vi "SpectrometerSpinCoater_v04_BetterStreaming.vi"() -> ()   [LabVIEW 2018]
uses:
  <instrlib>/Classes/CCD/Abstract_CCD/Abstract_CCD.lvclass
  TypDef/DeviceQueue_TypeDef.ctl
  TypDef/DeviceQueue_Action.ctl
  TypDef/DataQueue_TypeDef.ctl
  TypDef/DataQueue_Action.ctl
  <vilib>/Utility/error.llb/DialogType.ctl
  <instrlib>/Classes/CCD/Avantes/Avantes.lvclass
  C:/Program Files/National Instruments/LabVIEW 2018/instr.lib/Classes/CCD/Abstract_CCD/Abstract_CCD.lvclass
  <vilib>/Instr/_visa.llb/VISA Configure Serial Port (Instr).vi
panel:
  out "Time.spin":refnum<file>
  out "Meas.spin":refnum<file>
  out "Arduino":bool
  out "NKT":bool
  out "Spectromter":bool
  in  "Abort Button":bool
  in  "Stop Button":bool
  in  "Tab Control":enum32{"Measure", "Settings"}(tab)=enum."Settings"
  out "Action":string
  in  "Preview":bool
  out "XY Graph":T1(graph)
  in  "Frames for Dark/Ref":dbl=1.0
  in  "StartSpin_Button":bool
  out "Overall Time":dbl
  in  "Seconds after Spin Stop":dbl[unit]=0.5
  in  "Program Spin Coater\nSpeed (rpm)          Time (s)":dbl[][](array[numeric])
  in  "Record RefSpec":bool
  in  "Record_Darkspec":bool
  in  "Comments":string="Just for testing"
  in  "File Name":string="Temp"
  in  "Save Path":path=path "C:/Users/Timo/Desktop/SpinCoater/Measurement"
  in  "Seconds to Spin Start":dbl[unit]=1.0
  in  "Calculate Frames":bool=TRUE
  in  "Frames":i32
  out "Frame Rate":dbl[unit]
  in  "Integration Time":dbl[unit]=3e-05
  in  "StartMeasurement_Button":bool
  in  "Speed":dbl
  in  "Milliseconds":dbl
  in  "Debug":bool
  in  "Port Arduino":refnum<visa-resource-name>="COM6"
  out "Error Arduino":bool caption="Error"
  in  "Init_Arduino":bool=TRUE caption="Init"
  out "Caption_Settings_Arduino":string="Arduino"
  out "Caption_Settings_NKT":string="NKT Laser"
  out "Error_Spectromter":bool caption="Error"
  in  "Init_Spectrometer":bool=TRUE caption="Init"
  out "Caption_Settings_Spectrometer":string="Spectromter"
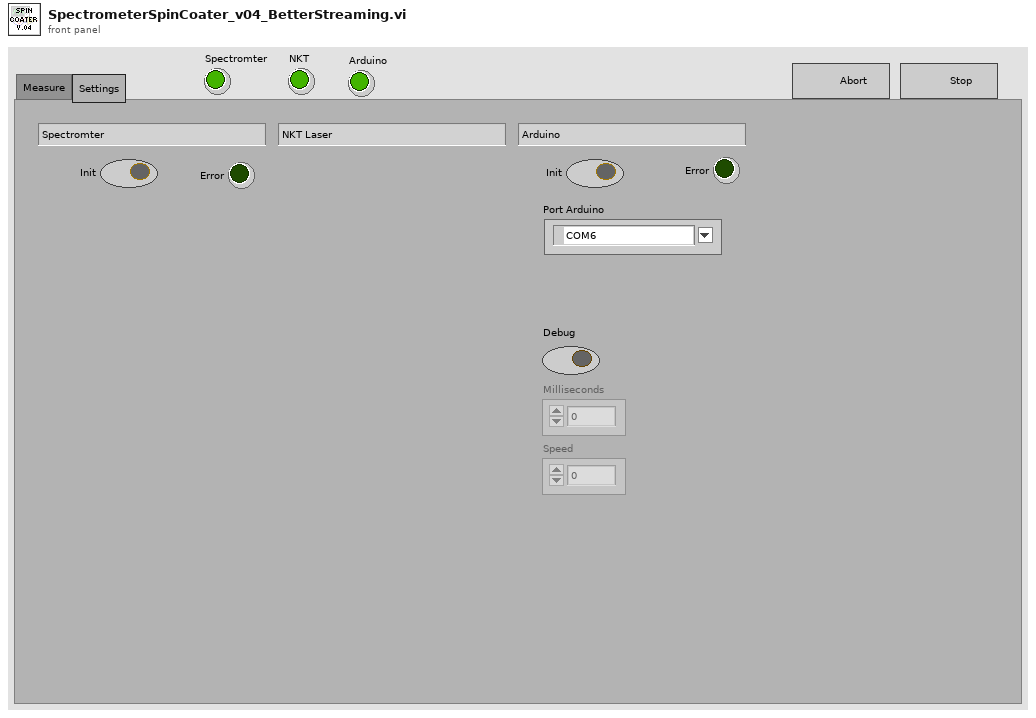
[diagram p1: front panel]
types:
  T1 = cluster{"Wavlength":dbl[unit][], "Image":dbl[]}[]
  T2 = cluster{"Dark":cluster{"Image":dbl[][][], "Frame Size":cluster{"F":i32, "Y":i32, "X":i32}}[], "Ref":cluster{"Image":dbl[][][], "Frame Size":cluster{"F":i32, "Y":i32, "X":i32}}[], "Wavlength":dbl[unit][], "spec":dbl[][]}
  T3 = cluster{"Port Arduino":refnum<visa-resource-name>, "Abstract_CCD.lvclass":refnum<class "Abstract_CCD.lvclass">}
  T4 = typedef "DataQueue_TypeDef.ctl" = cluster{"QueueAction":T5, "Data":cluster{"Image":dbl[][][], "Frame Size":cluster{"F":i32, "Y":i32, "X":i32}}[], "Data_Raw":cluster{"Image":dbl[][][], "Frame Size":cluster{"F":i32, "Y":i32, "X":i32}}[], "Data_Dark":cluster{"Image":dbl[][][], "Frame Size":cluster{"F":i32, "Y":i32, "X":i32}}[], "Data_Ref":cluster{"Image":dbl[][][], "Frame Size":cluster{"F":i32, "Y":i32, "X":i32}}[], "Device Information":string[], "Numeric Control":dbl, "Boolean":bool, "Wavelength":dbl[unit][], "Time":dbl[], "Time Stamp":timestamp, "Numeric Control 2":dbl}
  T5 = typedef "DataQueue_Action.ctl" = enum16{"TimeOut", "Close_Program", "Stop_Measurement", "Measure_InSituSpinCoating", "Save_Data", "Set_Ref", "Set_Dark", "Set_Wavelength", "Spectrometer_Measure", "Transfer_Settings"}
  T6 = typedef "DeviceQueue_TypeDef.ctl" = cluster{"QueueAction":T7, "Numeric 1":dbl, "Numeric 2":dbl, "Boolean 1":bool, "Boolean 2":bool, "Spin Program":dbl[][]}
  T7 = typedef "DeviceQueue_Action.ctl" = enum16{"TimeOut", "Close_Program", "Abort", "Spectrometer_Init", "Spectrometer_Close", "Spectrometer_DeviceInformation", "Spectrometer_Measure", "Spectrometer_Preview", "Spectrometer_Abort", "Spectrometer_StartMeasurement", "Spectrometer_GetData", "Spectrometer_StopMeasurement", "Spectrometer_SetIntegrationTime", "Spectrometer_SetFrames", "Spectrometer_SetDarkspec", "Spectrometer_SetReference", "Spectrometer_SetTriggerMode", "Laser_Init", "Laser_Close", "Arduino_Init", "Arduino_Close", "Arduino_LoadProgram", "Arduino_StartProgram", "Arduino_SetSpeed", "Arduino_SetMillis", "Arduino_StopSpin", "Measure_InSitu", "Measure_Stop"}
  T8 = enum16{"open", "replace", "create", "open or create", "replace or create", "replace or create with confirmation"}
  T9 = cluster{"Image":dbl[][][], "Frame Size":cluster{"F":i32, "Y":i32, "X":i32}}[]
  T10 = cluster{"Image":dbl[][][], "Frame Size":cluster{"F":i32, "Y":i32, "X":i32}}
  T11 = cluster{"Image":dbl[], "Image":dbl[], dbl[], "Numeric Control":dbl, "Numeric Control 2":dbl}
  T12 = typedef "DialogType.ctl" = u16
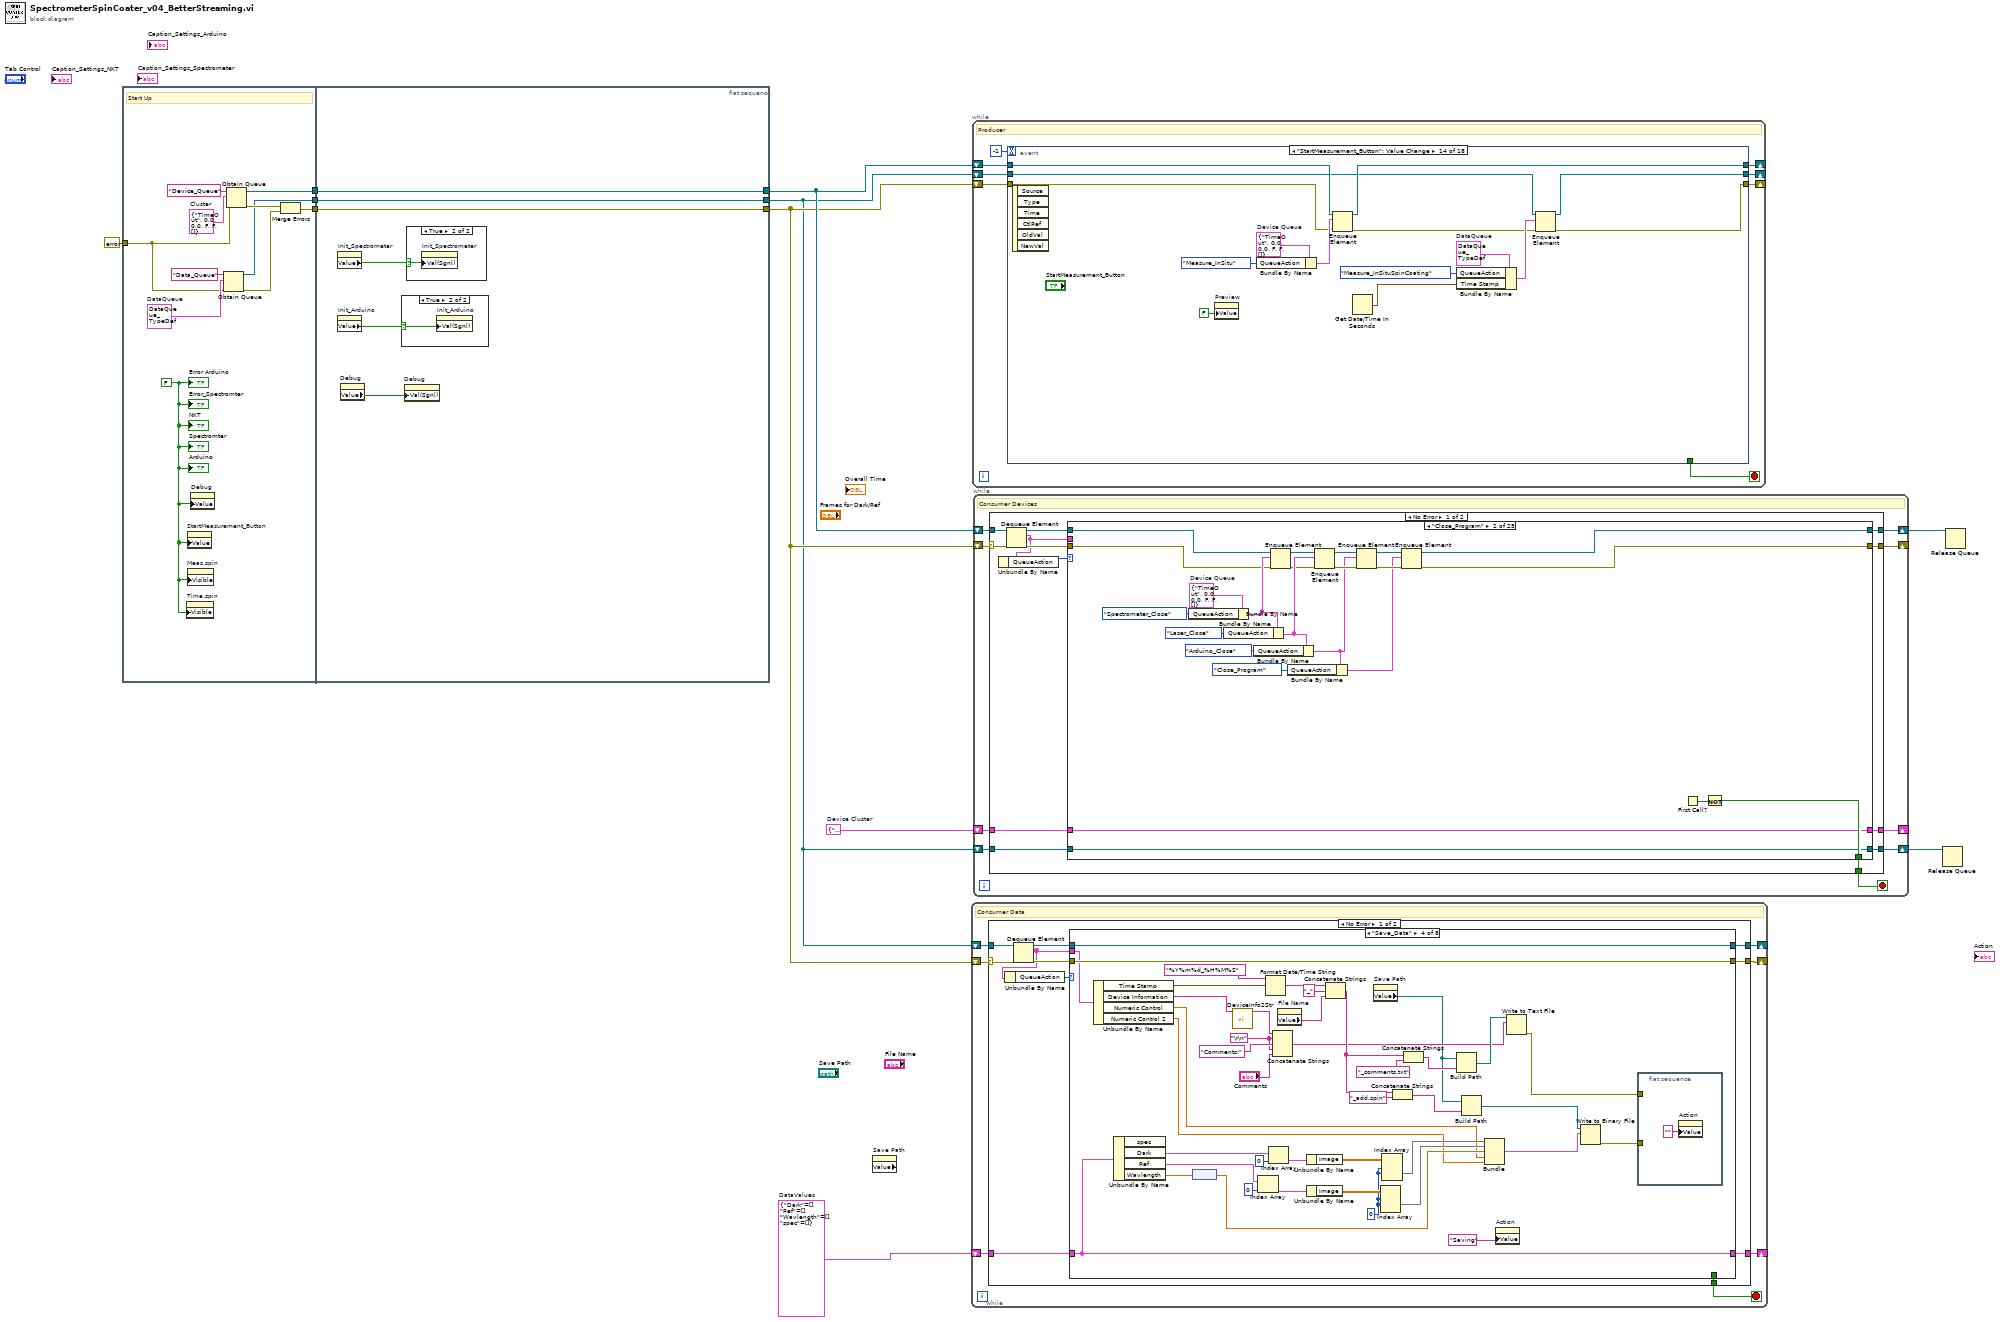
[diagram p0: block diagram]
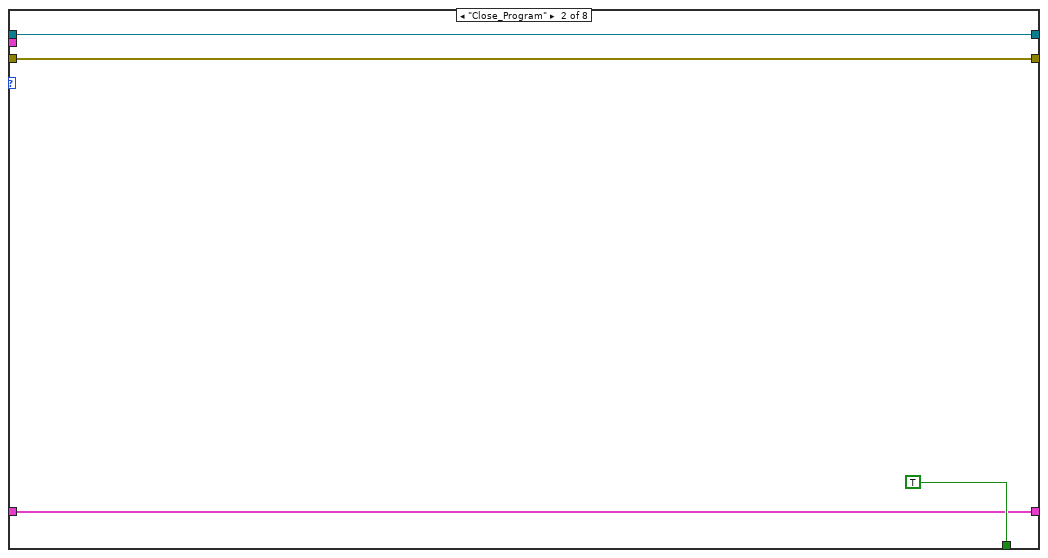
[diagram p5: hidden frame]
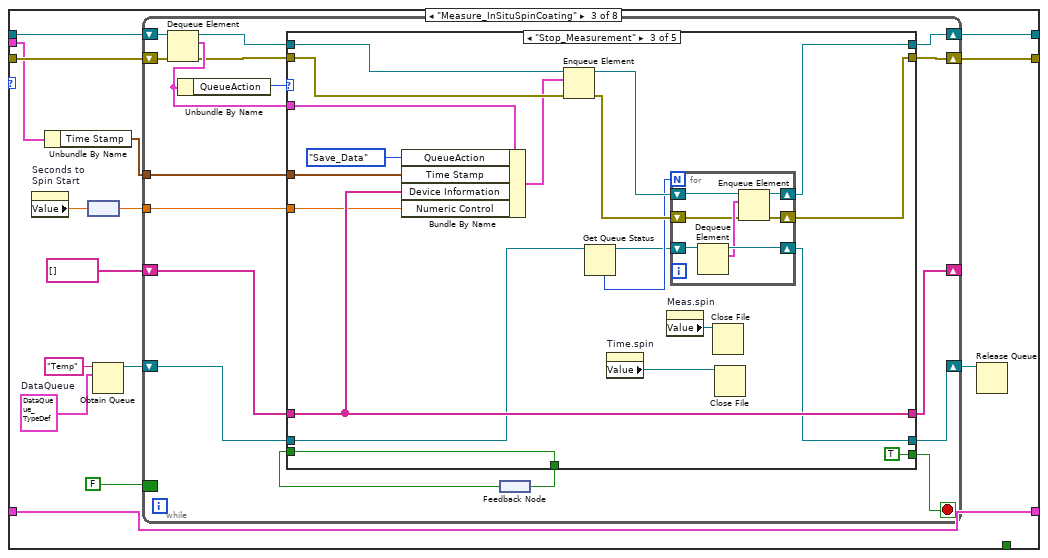
[diagram p6: hidden frame]
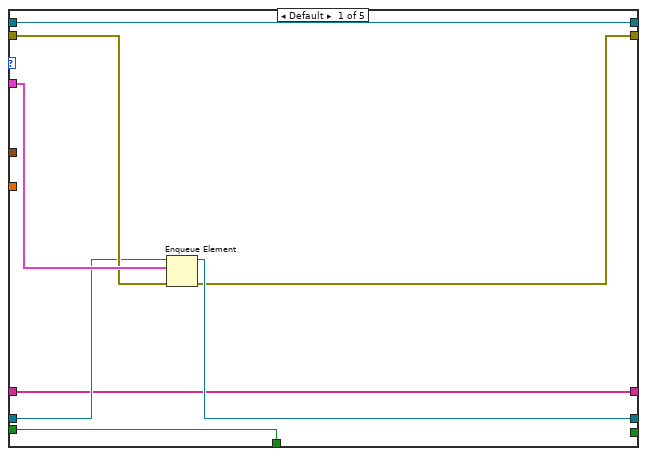
[diagram p7: hidden frame]
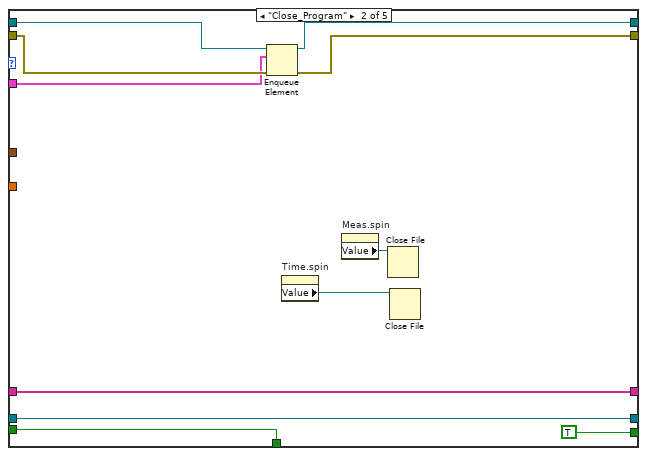
[diagram p8: hidden frame]
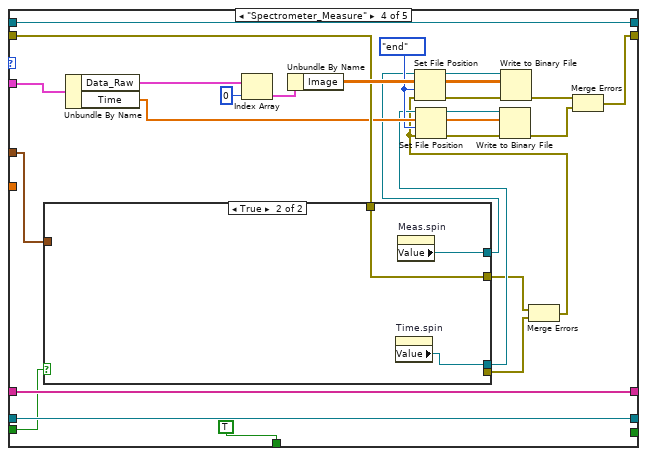
[diagram p9: hidden frame]
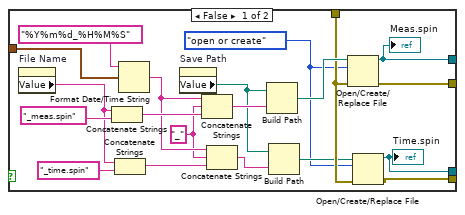
[diagram p10: hidden frame]
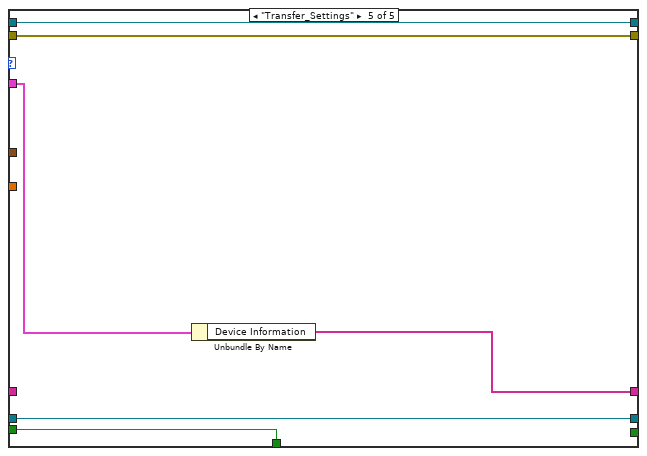
[diagram p11: hidden frame]
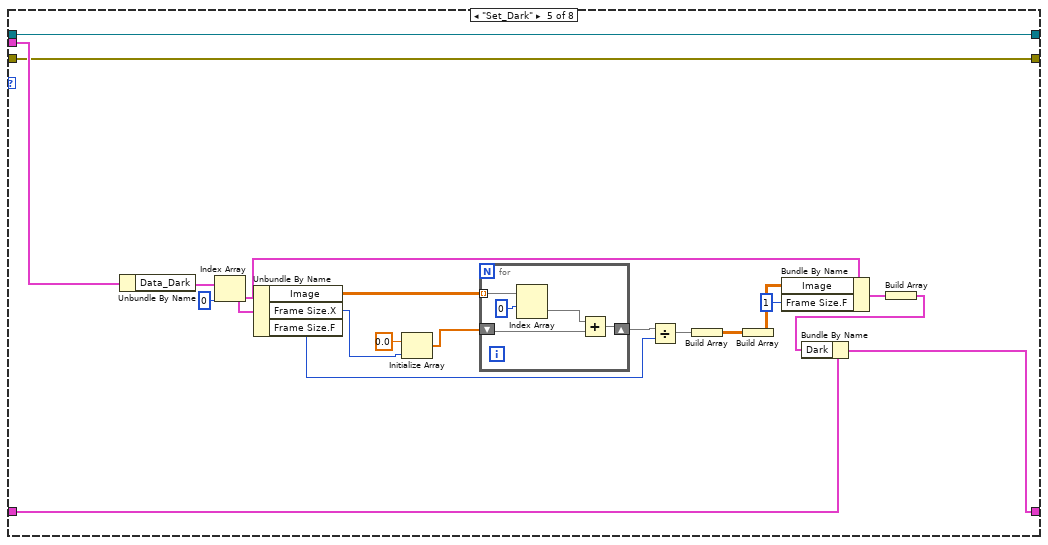
[diagram p12: hidden frame]
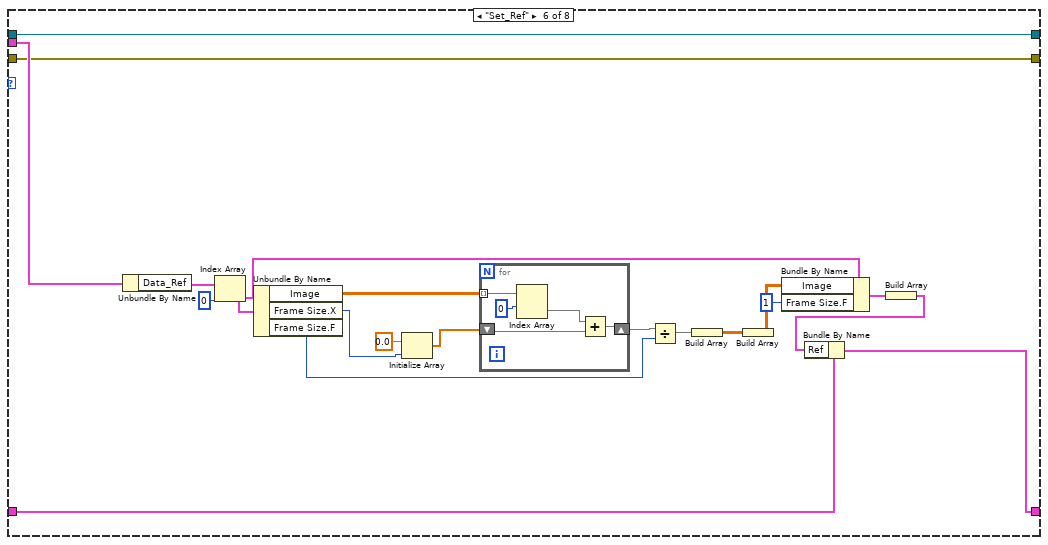
[diagram p13: hidden frame]
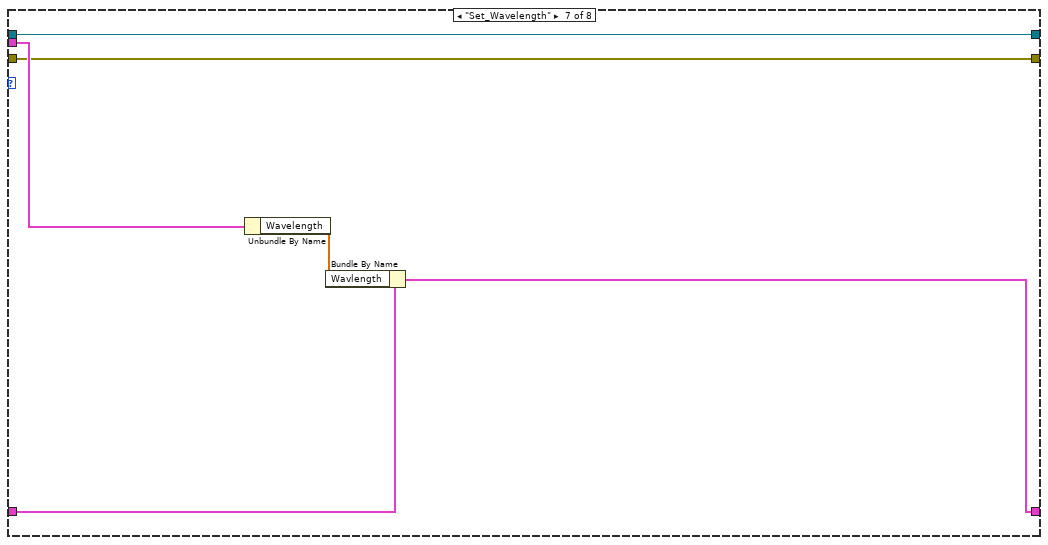
[diagram p14: hidden frame]
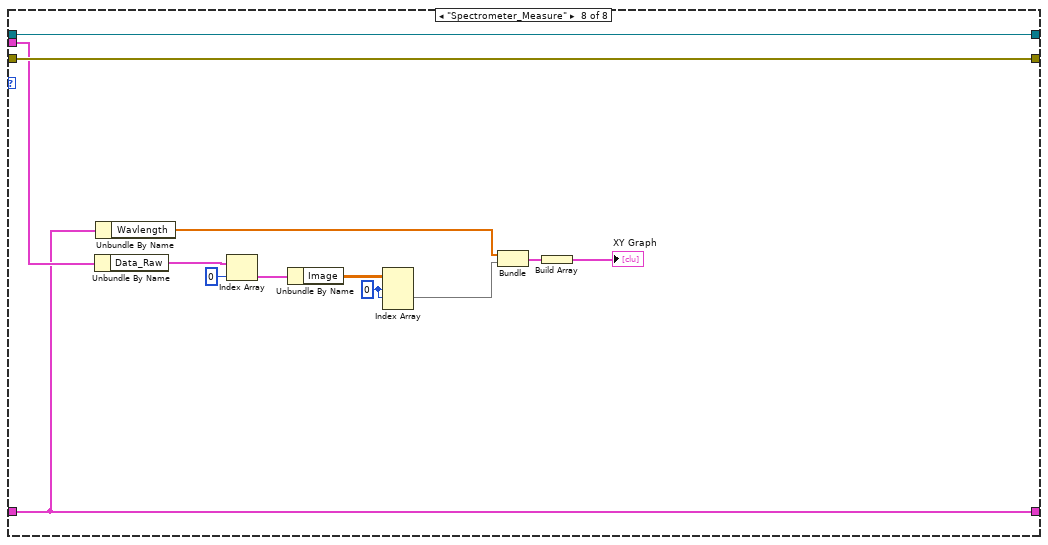
[diagram p15: hidden frame]
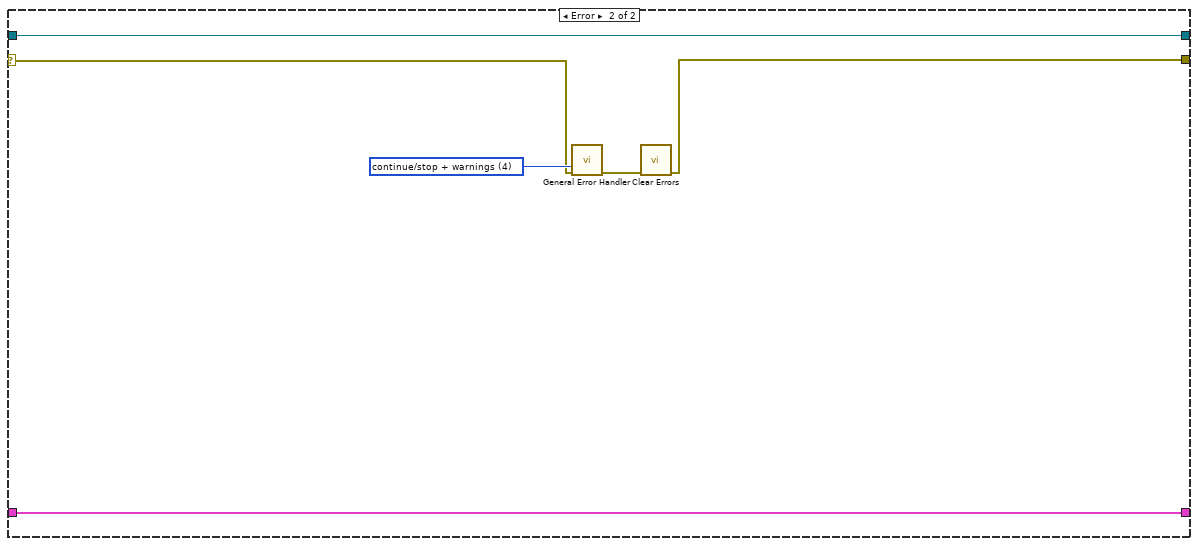
[diagram p16: hidden frame]
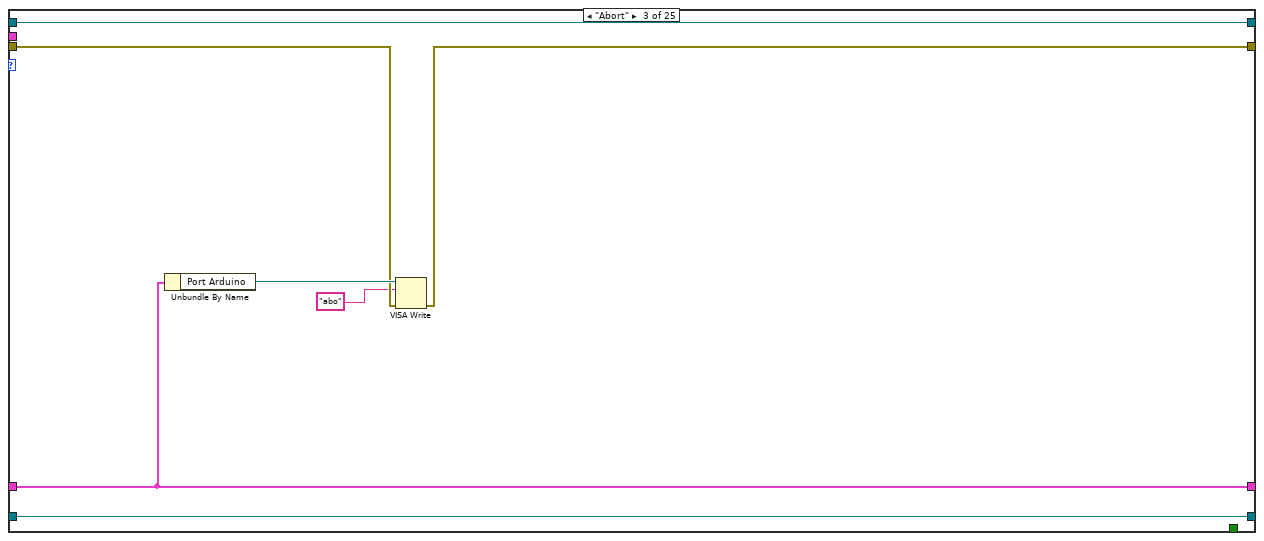
[diagram p18: hidden frame]
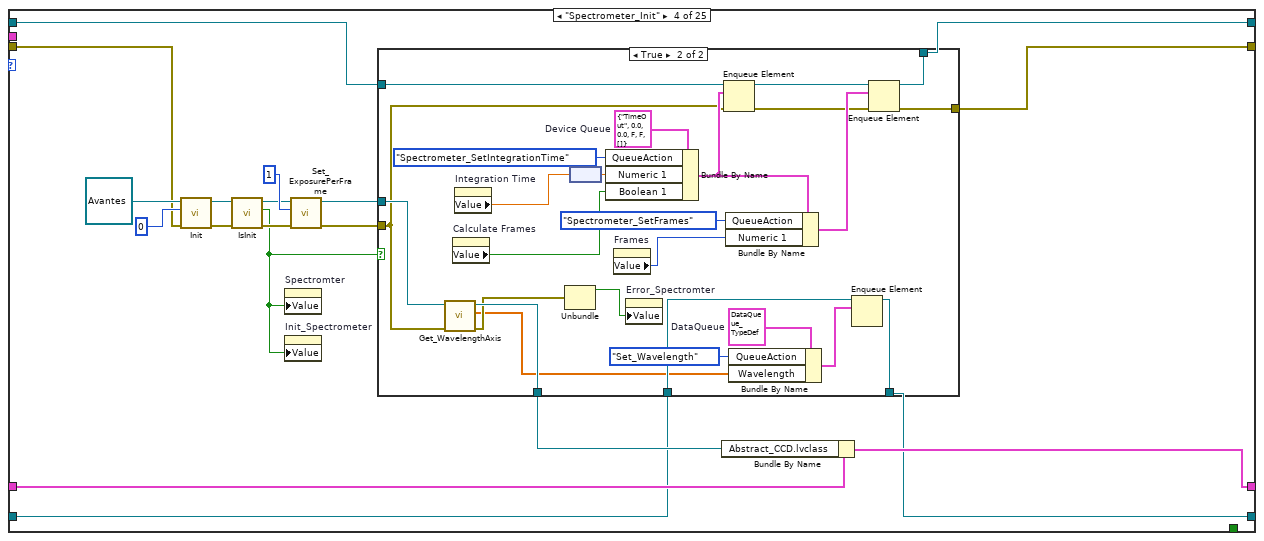
[diagram p19: hidden frame]
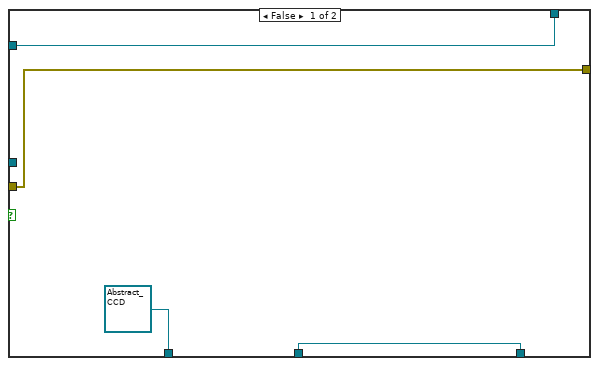
[diagram p20: hidden frame]
diagram:
  w1 = T2 {"Dark"=[], "Ref"=[], "Wavlength"=[], "spec"=[]}  # DataValues
  w6 = T3 {"Port Arduino"="", "Abstract_CCD.lvclass"=refnum}  # Device Cluster
  n1 = flat-sequence {
    tunnel: errorcluster {"status"=FALSE, "code"=0, "source"=""} ("error constant") -> [w17]
    tunnel: [w20] -> w10
    tunnel: [w14] -> w9
    tunnel: [w13] -> w8
    tunnel: w10 -> [w26]
    tunnel: w9 -> [w25]
    tunnel: w8 -> [w24]
    tunnel: [w26] -> w7
    tunnel: [w25] -> w2
    tunnel: [w24] -> w3
    frame #0 {
      w18 = T4 {"QueueAction"=enum."TimeOut", "Data"=[], "Data_Raw"=[], "Data_Dark"=[], "Data_Ref"=[], "Device Information"=[], "Numeric Control"=0.0, "Boolean"=FALSE, "Wavelength"=[], "Time"=[], "Time Stamp"=timestamp(0 s since 1904-01-01), "Numeric Control 2"=0.0}  # DataQueue
      w21 = T6 {"QueueAction"=enum."TimeOut", "Numeric 1"=0.0, "Numeric 2"=0.0, "Boolean 1"=FALSE, "Boolean 2"=FALSE, "Spin Program"=[]}  # Cluster
      w12 = FALSE ("Error Arduino")
      # "Start Up"
      n2 = property on="Time.spin" class="Ref (strict)"("Visible"=w12) -> ()  [unwired: 2 in, 2 out]
      n3 = property on="StartMeasurement_Button" class="Bool (strict)"("Value"=w12) -> ()  [unwired: 2 in, 2 out]
      n4 = property on="Meas.spin" class="Ref (strict)"("Visible"=w12) -> ()  [unwired: 2 in, 2 out]
      n5 = property on="Debug" class="Bool (strict)"("Value"=w12) -> ()  [unwired: 2 in, 2 out]
      n6 = Obtain Queue(name (unnamed)="Data_Queue", element data type=w18, error in (no error)=w17) -> (queue out=w14:refnum<queue>, error out=w15:errorcluster)  [unwired: 2 in, 1 out]
      n7 = Obtain Queue(name (unnamed)="Device_Queue", element data type=w21, error in (no error)=w17) -> (queue out=w20:refnum<queue>, error out=w16:errorcluster)  [unwired: 2 in, 1 out]
      n8 = Merge Errors(w16, w15) -> (w13:errorcluster)
      "Error_Spectromter" <- w12
      "Error Arduino" <- w12
      "Spectromter" <- w12
      "NKT" <- w12
      "Arduino" <- w12
    }
    frame #1 {
      n9 = property on="Init_Spectrometer" class="Bool (strict)"() -> ("Value"=w28:bool)  [unwired: 2 in, 2 out]
      n10 = property on="Init_Arduino" class="Bool (strict)"() -> ("Value"=w27:bool)  [unwired: 2 in, 2 out]
      n11 = property on="Debug" class="Bool (strict)"() -> ("Value"=w23:bool)  [unwired: 2 in, 2 out]
      n12 = case shown="True" w27 {
        selector: w27 -> [_ w29]
        frame False {
        }
        frame True {
          n13 = property on="Init_Arduino" class="Bool (strict)"("Val(Sgnl)"=w29) -> ()  [unwired: 2 in, 2 out]
        }
      }
      n14 = property on="Debug" class="Bool (strict)"("Val(Sgnl)"=w23) -> ()  [unwired: 2 in, 2 out]
      n15 = case shown="True" w28 {
        selector: w28 -> [_ w30]
        frame False {
        }
        frame True {
          n16 = property on="Init_Spectrometer" class="Bool (strict)"("Val(Sgnl)"=w30) -> ()  [unwired: 2 in, 2 out]
        }
      }
    }
  }
  n17 = property on="Save Path" class="Path" props=["Value"]() -> ()  [unwired: 2 in, 3 out]
  n18 = while {
    shift-right: [w31] -> _
    shift-left: w3 -> [w37]
    shift-right: [w32] -> _
    shift-left: w2 -> [w36]
    shift-right: [w33] -> _
    shift-left: w1 -> [w35]
    stop <- w34 stop-if-true
    # "Consumer Data"
    n19 = case shown="No Error" w37 {
      selector: w37 -> [w48 w303]
      tunnel: w36 -> [w47 w304]
      tunnel: w35 -> [w45 w301]
      tunnel: [w44 _] -> w34
      tunnel: [w43 w301] -> w33
      tunnel: [w42 w304] -> w32
      tunnel: [w40 w302] -> w31
      frame No Error {
        n20 = Dequeue Element(queue=w47, error in (no error)=w48) -> (queue out=w41:refnum<queue>, element=w38:T4, error out=w39:errorcluster)  [unwired: 1 in, 1 out]
        n21 = Unbundle By Name(w38) -> ("QueueAction"=w46:T5)
        n22 = case shown="\"Save_Data\"" w46 {
          tunnel: w45 -> [w49 w54 w60 w199 w251 w276 w286 w297]
          tunnel: [_ TRUE _ _ _ _ _ _] -> w44
          tunnel: [w49 w54 w60 w199 w247 w272 w285 w297] -> w43
          tunnel: [w51 w53 w70 w230 w248 w273 w282 w300] -> w42
          tunnel: w41 -> [w51 w53 w68 w230 w248 w273 w282 w300]
          tunnel: [w50 w52 w69 w229 w249 w274 w283 w299] -> w40
          tunnel: w39 -> [w50 w52 w67 w229 w249 w274 w283 w299]
          tunnel: w38 -> [_ _ w62 w215 w250 w275 w284 w298]
          frame "TimeOut", Default {
          }
          frame "Close_Program" {
          }
          frame "Measure_InSituSpinCoating" {
            w65 = T4 {"QueueAction"=enum."TimeOut", "Data"=[], "Data_Raw"=[], "Data_Dark"=[], "Data_Ref"=[], "Device Information"=[], "Numeric Control"=0.0, "Boolean"=FALSE, "Wavelength"=[], "Time"=[], "Time Stamp"=timestamp(0 s since 1904-01-01), "Numeric Control 2"=0.0}  # DataQueue
            n23 = property on="Seconds to\nSpin Start" class="DigNum (strict)"() -> ("Value"=w57:dbl[unit])  [unwired: 2 in, 2 out]
            n24 = Unbundle By Name(w62) -> ("Time Stamp"=w61:timestamp)
            n25 = node(w57) -> (w56:dbl)
            n26 = Obtain Queue(name (unnamed)="Temp", element data type=w65) -> (queue out=w64:refnum<queue>)  [unwired: 3 in, 2 out]
            n27 = while {
              shift-right: [w78] -> w70
              shift-left: w68 -> [w87]
              shift-right: [w79] -> w69
              shift-left: w67 -> [w86]
              shift-right: [w80] -> w63
              shift-left: w64 -> [w81]
              tunnel: w61 -> [w74]
              shift-right: [w75] -> _
              shift-left: string[] [] ("Device Information") -> [w76]
              border: FALSE -> [_]
              tunnel: w56 -> [w71]
              stop <- w77 stop-if-true
              n28 = Dequeue Element(queue=w87, error in (no error)=w86) -> (queue out=w82:refnum<queue>, element=w84:T4, error out=w83:errorcluster)  [unwired: 1 in, 1 out]
              n29 = Unbundle By Name(w84) -> ("QueueAction"=w85:T5)
              n30 = feedback #1() -> (w73:bool)
              n31 = case shown="\"Stop_Measurement\"" w85 {
                tunnel: w84 -> [w95 w104 w125 w158 w187]
                tunnel: w83 -> [w94 w105 w122 w148 w184]
                tunnel: w82 -> [w90 w106 w121 w157 w185]
                tunnel: w81 -> [w93 w101 w116 w145 w188]
                tunnel: [w92 w101 w113 w145 w188] -> w80
                tunnel: [w91 w102 w112 w146 w184] -> w79
                tunnel: [w90 w103 w111 w157 w185] -> w78
                tunnel: [_ TRUE TRUE _ _] -> w77
                tunnel: w76 -> [w89 w99 w123 w143 _]
                tunnel: [w89 w99 w123 w143 w186] -> w75
                tunnel: w74 -> [_ _ w124 w159 _]
                tunnel: w73 -> [w88 w98 w110 w141 w183]
                tunnel: [w88 w98 w110 TRUE w183] -> w72
                tunnel: w71 -> [_ _ w107 _ _]
                frame Default {
                  n32 = Enqueue Element(queue=w93, element=w95, error in (no error)=w94) -> (queue out=w92:refnum<queue>, error out=w91:errorcluster)  [unwired: 1 in, 1 out]
                }
                frame "Close_Program" {
                  n33 = Enqueue Element(queue=w106, element=w104, error in (no error)=w105) -> (queue out=w103:refnum<queue>, error out=w102:errorcluster)  [unwired: 1 in, 1 out]
                  n34 = property on="Time.spin" class="Ref (strict)"() -> ("Value"=w96:refnum<file>)  [unwired: 2 in, 2 out]
                  n35 = property on="Meas.spin" class="Ref (strict)"() -> ("Value"=w97:refnum<file>)  [unwired: 2 in, 2 out]
                  n36 = Close File(refnum=w97) -> ()  [unwired: 1 in, 2 out]
                  n37 = Close File(refnum=w96) -> ()  [unwired: 1 in, 2 out]
                }
                frame "Stop_Measurement" {
                  n38 = Bundle By Name(cluster=w125, "QueueAction"=DataQueue_Action."Save_Data", "Time Stamp"=w124, "Device Information"=w123, "Numeric Control"=w107) -> (w120:T4)
                  n39 = Enqueue Element(queue=w121, element=w120, error in (no error)=w122) -> (queue out=w118:refnum<queue>, error out=w117:errorcluster)  [unwired: 1 in, 1 out]
                  n40 = Get Queue Status(queue=w116) -> (queue out=w114:refnum<queue>, # elements in queue=w115:i32)  [unwired: 2 in, 6 out]
                  n41 = property on="Time.spin" class="Ref (strict)"() -> ("Value"=w108:refnum<file>)  [unwired: 2 in, 2 out]
                  n42 = property on="Meas.spin" class="Ref (strict)"() -> ("Value"=w109:refnum<file>)  [unwired: 2 in, 2 out]
                  n43 = for {
                    N: w115 -> [_]
                    shift-right: [w132] -> w113
                    shift-left: w114 -> [w133]
                    shift-right: [w129] -> w111
                    shift-left: w118 -> [w130]
                    shift-right: [w127] -> w112
                    shift-left: w117 -> [w128]
                    n44 = Dequeue Element(queue=w133) -> (queue out=w132:refnum<queue>, element=w131:T4)  [unwired: 2 in, 2 out]
                    n45 = Enqueue Element(queue=w130, element=w131, error in (no error)=w128) -> (queue out=w129:refnum<queue>, error out=w127:errorcluster)  [unwired: 1 in, 1 out]
                  }
                  n46 = Close File(refnum=w109) -> ()  [unwired: 1 in, 2 out]
                  n47 = Close File(refnum=w108) -> ()  [unwired: 1 in, 2 out]
                }
                frame "Spectrometer_Measure" {
                  w144 = enum16{"start", "end", "current"}."end" ("from (0:start)")
                  n48 = case shown="True" w141 {
                    tunnel: w159 -> [w176 _]
                    tunnel: w148 -> [w171 w182]
                    tunnel: [w164 w182] -> w135
                    tunnel: [w163 _] -> w136
                    tunnel: [w162 w181] -> w138
                    tunnel: [w161 w180] -> w137
                    frame False {
                      w165 = T8."open or create" ("operation (0:open)")
                      w160 = "_" ("string")
                      n49 = property on="File Name" class="Str"() -> ("Value"=w174:string)  [unwired: 2 in, 2 out]
                      n50 = Concatenate Strings(w174, "_meas.spin" ("string")) -> (w177:string)
                      n51 = Concatenate Strings(w174, "_time.spin" ("string")) -> (w169:string)
                      n52 = Format Date/Time String(time format string (%c)="%Y%m%d_%H%M%S", seconds (now)=w176) -> (date/time string=w170:string)  [unwired: 1 in]
                      n53 = property on="Save Path" class="Path"() -> ("Value"=w167:path)  [unwired: 2 in, 2 out]
                      n54 = Concatenate Strings(w170, w160, w177) -> (w175:string)
                      n55 = Concatenate Strings(w170, w160, w169) -> (w168:string)
                      n56 = Build Path(base path=w167, name or relative path=w175) -> (appended path=w172:path)
                      n57 = Build Path(base path=w167, name or relative path=w168) -> (appended path=w166:path)
                      n58 = Open/Create/Replace File(file path (use dialog)=w172, error in=w171, operation (0:open)=w165) -> (refnum out=w162:refnum<file>, error out=w164:errorcluster)  [unwired: 3 in, 1 out]
                      "Meas.spin" <- w162
                      n59 = Open/Create/Replace File(file path (use dialog)=w166, error in=w171, operation (0:open)=w165) -> (refnum out=w161:refnum<file>, error out=w163:errorcluster)  [unwired: 3 in, 1 out]
                      "Time.spin" <- w161
                    }
                    frame True {
                      n60 = property on="Time.spin" class="Ref (strict)"() -> ("Value"=w180:refnum<file>)  [unwired: 2 in, 2 out]
                      n61 = property on="Meas.spin" class="Ref (strict)"() -> ("Value"=w181:refnum<file>)  [unwired: 2 in, 2 out]
                    }
                  }
                  n62 = Unbundle By Name(w158) -> ("Data_Raw"=w154:T9, "Time"=w147:dbl[])
                  n63 = Index Array(array=w154, index=0) -> (element=w153:T10)
                  n64 = Unbundle By Name(w153) -> ("Image"=w151:dbl[][][])
                  n65 = Merge Errors(w135, w136) -> (w134:errorcluster)
                  n66 = Set File Position(refnum=w138, from (0:start)=w144, error in=w134) -> (refnum out=w150:refnum<file>, error out=w149:errorcluster)  [unwired: 1 in]
                  n67 = Set File Position(refnum=w137, from (0:start)=w144, error in=w134) -> (refnum out=w156:refnum<file>, error out=w155:errorcluster)  [unwired: 1 in]
                  n68 = Write to Binary File(file (use dialog)=w156, data=w147, error in=w155) -> (error out=w139:errorcluster)  [unwired: 3 in, 2 out]
                  n69 = Write to Binary File(file (use dialog)=w150, data=w151, error in=w149) -> (error out=w140:errorcluster)  [unwired: 3 in, 2 out]
                  n70 = Merge Errors(w140, w139) -> (w146:errorcluster)
                }
                frame "Transfer_Settings" {
                  n71 = Unbundle By Name(w187) -> ("Device Information"=w186:string[])
                }
              }
              n72 = feedback-in #1(w72) -> ()
            }
            n73 = Release Queue(queue=w63) -> ()  [unwired: 2 in, 3 out]
          }
          frame "Save_Data" {
            w201 = "\r\n"
            w219 = 0 ("index (page)")
            n74 = Unbundle By Name(w215) -> ("Time Stamp"=w213:timestamp, "Device Information"=w204:string[], "Numeric Control"=w198:dbl, "Numeric Control 2"=w197:dbl)
            n75 = Unbundle By Name(w199) -> ("Dark"=w226:T9, "Ref"=w224:T9, "Wavlength"=w228:dbl[unit][])  [unwired: 1 out]
            n76 = node(w228) -> (w216:dbl[])
            n77 = call "DeviceInfo2Str.vi"("Device Information"=w204) -> ("String"=w203:string)  [unwired: 10 in]
            n78 = Index Array(array=w224, index=0) -> (element=w222:T10)
            n79 = Format Date/Time String(time format string (%c)="%Y%m%d_%H%M%S", seconds (now)=w213) -> (date/time string=w212:string)  [unwired: 1 in]
            n80 = Index Array(array=w226, index=0) -> (element=w223:T10)
            n81 = Concatenate Strings(w203, w201, "Comments:" ("string"), w201, "Comments") -> (w196:string)
            n82 = property on="File Name" class="Str"() -> ("Value"=w194:string)  [unwired: 2 in, 2 out]
            n83 = Unbundle By Name(w223) -> ("Image"=w221:dbl[][][])
            n84 = Unbundle By Name(w222) -> ("Image"=w220:dbl[][][])
            n85 = Concatenate Strings(w212, "_" ("string"), w194) -> (w210:string)
            n86 = property on="Save Path" class="Path"() -> ("Value"=w193:path)  [unwired: 2 in, 2 out]
            n87 = Index Array(array=w220, index (dim 0)=w219, index (dim 1)=w219) -> (element=w217:dbl[])  [unwired: 1 in]
            n88 = Index Array(array=w221, index (dim 0)=w219, index (dim 1)=w219) -> (element=w218:dbl[])  [unwired: 1 in]
            n89 = Concatenate Strings(w210, "_add.spin" ("string")) -> (w208:string)
            n90 = Concatenate Strings(w210, "_comments.txt" ("string")) -> (w207:string)
            n91 = Build Path(base path=w193, name or relative path=w207) -> (appended path=w206:path)
            n92 = Build Path(base path=w193, name or relative path=w208) -> (appended path=w192:path)
            n93 = Bundle("Image"=w218, "Image"=w217, w216, "Numeric Control"=w198, "Numeric Control 2"=w197) -> (w191:T11)  [unwired: 1 in]
            n94 = property on="Action" class="Str"("Value"="Saving" ("Action")) -> ()  [unwired: 2 in, 2 out]
            n95 = Write to Text File(file (use dialog)=w206, text=w196) -> (error out=w190:errorcluster)  [unwired: 2 in, 2 out]
            n96 = Write to Binary File(file (use dialog)=w192, data=w191) -> (error out=w189:errorcluster)  [unwired: 4 in, 2 out]
            n97 = flat-sequence {
              tunnel: w190 -> [_]
              tunnel: w189 -> [_]
              frame #0 {
                n98 = property on="Action" class="Str"("Value"="" ("Action")) -> ()  [unwired: 2 in, 2 out]
              }
            }
          }
          frame "Set_Dark" {
            n99 = Unbundle By Name(w250) -> ("Data_Dark"=w237:T9)
            n100 = Index Array(array=w237, index=0) -> (element=w236:T10)
            n101 = Unbundle By Name(w236) -> ("Image"=w245:dbl[][][], "Frame Size.X"=w243:i32, "Frame Size.F"=w240:i32)
            n102 = Initialize Array(0.0 ("element"), w243) -> (w242:dbl[])
            n103 = for {
              tunnel: w245 -> [w256] mode=indexing
              shift-right: [w252] -> w241
              shift-left: w242 -> [w253]
              n104 = Index Array(array=w256, index (row)=0) -> (element=w254:dbl[])  [unwired: 1 in]
              n105 = Add(x=w254, y=w253) -> (x+y=w252:dbl[])
            }
            n106 = Divide(x=w241, y=w240) -> (x/y=w239:dbl[])
            n107 = Build Array(w239) -> (w238:dbl[][])
            n108 = Build Array(w238) -> (w235:dbl[][][])
            n109 = Bundle By Name(cluster=w236, "Image"=w235, "Frame Size.F"=1) -> (w233:T10)
            n110 = Build Array(w233) -> (w232:T9)
            n111 = Bundle By Name(cluster=w251, "Dark"=w232) -> (w247:T2)
          }
          frame "Set_Ref" {
            n112 = Unbundle By Name(w275) -> ("Data_Ref"=w262:T9)
            n113 = Index Array(array=w262, index=0) -> (element=w261:T10)
            n114 = Unbundle By Name(w261) -> ("Image"=w270:dbl[][][], "Frame Size.X"=w268:i32, "Frame Size.F"=w265:i32)
            n115 = Initialize Array(0.0 ("element"), w268) -> (w267:dbl[])
            n116 = for {
              tunnel: w270 -> [w281] mode=indexing
              shift-right: [w277] -> w266
              shift-left: w267 -> [w278]
              n117 = Index Array(array=w281, index (row)=0) -> (element=w279:dbl[])  [unwired: 1 in]
              n118 = Add(x=w279, y=w278) -> (x+y=w277:dbl[])
            }
            n119 = Divide(x=w266, y=w265) -> (x/y=w264:dbl[])
            n120 = Build Array(w264) -> (w263:dbl[][])
            n121 = Build Array(w263) -> (w260:dbl[][][])
            n122 = Bundle By Name(cluster=w261, "Image"=w260, "Frame Size.F"=1) -> (w258:T10)
            n123 = Build Array(w258) -> (w257:T9)
            n124 = Bundle By Name(cluster=w276, "Ref"=w257) -> (w272:T2)
          }
          frame "Set_Wavelength" {
            n125 = Unbundle By Name(w284) -> ("Wavelength"=w287:dbl[unit][])
            n126 = Bundle By Name(cluster=w286, "Wavlength"=w287) -> (w285:T2)
          }
          frame "Spectrometer_Measure" {
            w292 = 0 ("index (page)")
            n127 = Unbundle By Name(w298) -> ("Data_Raw"=w296:T9)
            n128 = Unbundle By Name(w297) -> ("Wavlength"=w291:dbl[unit][])
            n129 = Index Array(array=w296, index=0) -> (element=w294:T10)
            n130 = Unbundle By Name(w294) -> ("Image"=w293:dbl[][][])
            n131 = Index Array(array=w293, index (dim 0)=w292, index (dim 1)=w292) -> (element=w290:dbl[])  [unwired: 1 in]
            n132 = Bundle("Wavlength"=w291, "Image"=w290) -> (w289:cluster{"Wavlength":dbl[unit][], "Image":dbl[]})  [unwired: 1 in]
            n133 = Build Array(w289) -> (→"XY Graph":T1)
          }
        }
      }
      frame Error {
        w306 = T12 4 items=["no dialog", "OK message", "continue or stop message", "OK message + warnings", "continue/stop + warnings"] ("type of dialog (OK msg:1)")
        n134 = call <vilib>:"General Error Handler.vi"("type of dialog (OK msg:1)"=w306, "error in (no error)"=w303) -> ("error out"=w305:errorcluster)  [unwired: 9 in, 4 out]
        n135 = call <vilib>:"Clear Errors.vi"("error in (no error)"=w305) -> ("error out"=w302:errorcluster)  [unwired: 5 in, 1 out]
      }
    }
  }
  n136 = while {
    shift-right: [w309] -> _
    shift-left: w7 -> [w307]
    shift-right: [w312] -> _
    shift-left: w2 -> [w313]
    shift-right: [w310] -> _
    shift-left: w3 -> [w311]
    stop <- w308 stop-if-true
    # "Producer"
    n137 = event shown="[13] \"StartMeasurement_Button\": Value Change" {
      selector: _ -> [_ _ _ _ _ _ _ _ _ _ _ _ _ _ _ _ _ _]
      dyn-events: _ -> [_ _ _ _ _ _ _ _ _ _ _ _ _ _ _ _ _ _]
      timeout: -1 -> [_ _ _ _ _ _ _ _ _ _ _ _ _ _ _ _ _ _]
      tunnel: w313 -> [w316 w331 w335 w347 w360 w375 w387 w398 w401 w408 w427 w434 w443 w451 w466 w476 w485 w493]
      tunnel: [w316 w328 w335 w347 w360 w375 w387 w398 w401 w408 w427 w434 w443 w450 w466 w476 w485 w493] -> w312
      tunnel: w311 -> [w315 w330 w337 w345 w357 w374 w385 w393 w400 w405 w425 w433 w441 w457 w463 w475 w484 w492]
      tunnel: [w315 w324 w334 w341 w356 w372 w383 w392 w400 w403 w424 w431 w440 w449 w464 w472 w481 w492] -> w310
      tunnel: w307 -> [w317 w332 w338 w346 w359 w376 w386 w395 w402 w406 w428 w435 w444 w459 w467 w477 w486 w494]
      tunnel: [w317 w329 w336 w342 w358 w373 w384 w394 w402 w407 w426 w432 w442 w458 w465 w473 w482 w494] -> w309
      tunnel: [_ TRUE _ _ _ _ _ _ _ _ _ _ _ _ _ _ _ _] -> w308
      event Timeout {
        n138 = event-data() -> ()  [unwired: 1 in, 3 out]
      }
      event "Stop Button": Value Change {
        w320 = T4 {"QueueAction"=enum."TimeOut", "Data"=[], "Data_Raw"=[], "Data_Dark"=[], "Data_Ref"=[], "Device Information"=[], "Numeric Control"=0.0, "Boolean"=FALSE, "Wavelength"=[], "Time"=[], "Time Stamp"=timestamp(0 s since 1904-01-01), "Numeric Control 2"=0.0}  # DataQueue
        w323 = T6 {"QueueAction"=enum."TimeOut", "Numeric 1"=0.0, "Numeric 2"=0.0, "Boolean 1"=FALSE, "Boolean 2"=FALSE, "Spin Program"=[]}  # Device Queue
        n139 = event-data() -> ()  [unwired: 1 in, 6 out]
        n140 = Bundle By Name(cluster=w323, "QueueAction"=DeviceQueue_Action."Close_Program") -> (w321:T6)
        n141 = Enqueue Element(queue=w332, element=w321, error in (no error)=w330) -> (queue out=w329:refnum<queue>, error out=w325:errorcluster)  [unwired: 1 in, 1 out]
        n142 = Bundle By Name(cluster=w320, "QueueAction"=DataQueue_Action."Close_Program") -> (w318:T4)
        n143 = Enqueue Element(queue=w331, element=w318, error in (no error)=w330) -> (queue out=w328:refnum<queue>, error out=w326:errorcluster)  [unwired: 1 in, 1 out]
        n144 = Merge Errors(w326, w325) -> (w324:errorcluster)
      }
      event "Abort Button": Value Change {
        w340 = T6 {"QueueAction"=enum."TimeOut", "Numeric 1"=0.0, "Numeric 2"=0.0, "Boolean 1"=FALSE, "Boolean 2"=FALSE, "Spin Program"=[]}  # Device Queue
        # "At the moment just spin coater in non in-situ measurements can be stopped"
        n145 = event-data() -> ()  [unwired: 1 in, 6 out]
        n146 = Bundle By Name(cluster=w340, "QueueAction"=DeviceQueue_Action."Abort") -> (w339:T6)
        n147 = Enqueue Element(queue=w338, element=w339, error in (no error)=w337) -> (queue out=w336:refnum<queue>, error out=w334:errorcluster)  [unwired: 1 in, 1 out]
      }
      event "Init_Spectrometer": Value Change {
        n148 = event-data() -> ()  [unwired: 1 in, 6 out]
        n149 = case shown="False" "Init_Spectrometer" {
          tunnel: [w348 w351] -> w343
          frame True {
            n150 = Bundle By Name(cluster=T6 {"QueueAction"=enum."TimeOut", "Numeric 1"=0.0, "Numeric 2"=0.0, "Boolean 1"=FALSE, "Boolean 2"=FALSE, "Spin Program"=[]} ("element"), "QueueAction"=DeviceQueue_Action."Spectrometer_Init") -> (w348:T6)
          }
          frame False {
            n151 = Bundle By Name(cluster=T6 {"QueueAction"=enum."TimeOut", "Numeric 1"=0.0, "Numeric 2"=0.0, "Boolean 1"=FALSE, "Boolean 2"=FALSE, "Spin Program"=[]} ("element"), "QueueAction"=DeviceQueue_Action."Spectrometer_Close") -> (w351:T6)
          }
        }
        n152 = Enqueue Element(queue=w346, element=w343, error in (no error)=w345) -> (queue out=w342:refnum<queue>, error out=w341:errorcluster)  [unwired: 1 in, 1 out]
      }
      event "Init_Arduino": Value Change {
        n153 = event-data() -> ("NewVal"=w355:bool)  [unwired: 1 in, 5 out]
        n154 = case shown="True" w355 {
          tunnel: [w361 w364] -> w354
          frame False {
            w363 = T6 {"QueueAction"=enum."TimeOut", "Numeric 1"=0.0, "Numeric 2"=0.0, "Boolean 1"=FALSE, "Boolean 2"=FALSE, "Spin Program"=[]}  # Device Queue
            n155 = Bundle By Name(cluster=w363, "QueueAction"=DeviceQueue_Action."Arduino_Close") -> (w361:T6)
          }
          frame True {
            w366 = T6 {"QueueAction"=enum."TimeOut", "Numeric 1"=0.0, "Numeric 2"=0.0, "Boolean 1"=FALSE, "Boolean 2"=FALSE, "Spin Program"=[]}  # Device Queue
            n156 = Bundle By Name(cluster=w366, "QueueAction"=DeviceQueue_Action."Arduino_Init") -> (w364:T6)
          }
        }
        n157 = Enqueue Element(queue=w359, element=w354, error in (no error)=w357) -> (queue out=w358:refnum<queue>, error out=w356:errorcluster)  [unwired: 1 in, 1 out]
      }
      event "Program Spin Coater\nSpeed (rpm)          Time (s)": Value Change {
        w378 = T6 {"QueueAction"=enum."TimeOut", "Numeric 1"=0.0, "Numeric 2"=0.0, "Boolean 1"=FALSE, "Boolean 2"=FALSE, "Spin Program"=[]}  # Device Queue
        n158 = event-data() -> ("NewVal"=w370:dbl[][])  [unwired: 1 in, 5 out]
        n159 = property on="Seconds to Spin Start" class="DigNum (strict)"() -> ("Value"=w368:dbl[unit])  [unwired: 2 in, 2 out]
        n160 = node(w368) -> (w367:dbl)
        n161 = Bundle By Name(cluster=w378, "QueueAction"=DeviceQueue_Action."Arduino_LoadProgram", "Spin Program"=w370, "Numeric 1"=w367) -> (w377:T6)
        n162 = Enqueue Element(queue=w376, element=w377, error in (no error)=w374) -> (queue out=w373:refnum<queue>, error out=w372:errorcluster)  [unwired: 1 in, 1 out]
        n163 = property on="Integration Time" class="DigNum (strict)"() -> ("Value"=w369:dbl[unit])  [unwired: 2 in, 2 out]
        n164 = property on="Integration Time" class="DigNum (strict)"("Val(Sgnl)"=w369) -> ()  [unwired: 2 in, 2 out]
      }
      event "Integration Time": Value Change {
        w389 = T6 {"QueueAction"=enum."TimeOut", "Numeric 1"=0.0, "Numeric 2"=0.0, "Boolean 1"=FALSE, "Boolean 2"=FALSE, "Spin Program"=[]}  # Device Queue
        n165 = event-data() -> ("NewVal"=w381:dbl[unit])  [unwired: 1 in, 5 out]
        n166 = node(w381) -> (w380:dbl)
        n167 = property on="Calculate Frames" class="Bool (strict)"() -> ("Value"=w379:bool)  [unwired: 2 in, 2 out]
        n168 = Bundle By Name(cluster=w389, "QueueAction"=DeviceQueue_Action."Spectrometer_SetIntegrationTime", "Numeric 1"=w380, "Boolean 1"=w379) -> (w388:T6)
        n169 = Enqueue Element(queue=w386, element=w388, error in (no error)=w385) -> (queue out=w384:refnum<queue>, error out=w383:errorcluster)  [unwired: 1 in, 1 out]
      }
      event "Frames": Value Change {
        w397 = T6 {"QueueAction"=enum."TimeOut", "Numeric 1"=0.0, "Numeric 2"=0.0, "Boolean 1"=FALSE, "Boolean 2"=FALSE, "Spin Program"=[]}  # Device Queue
        n170 = event-data() -> ()  [unwired: 1 in, 6 out]
        n171 = Bundle By Name(cluster=w397, "QueueAction"=DeviceQueue_Action."Spectrometer_SetFrames", "Numeric 1"="Frames") -> (w396:T6)
        n172 = Enqueue Element(queue=w395, element=w396, error in (no error)=w393) -> (queue out=w394:refnum<queue>, error out=w392:errorcluster)  [unwired: 1 in, 1 out]
      }
      event "Seconds to Spin Start", "Seconds after Spin Stop": Value Change {
        n173 = event-data() -> ()  [unwired: 1 in, 6 out]
        n174 = property on="Program Spin Coater\nSpeed (rpm)          Time (s)" class="Arr (strict)"() -> ("Value"=w399:dbl[][])  [unwired: 2 in, 2 out]
        n175 = property on="Program Spin Coater\nSpeed (rpm)          Time (s)" class="Arr (strict)"("Val(Sgnl)"=w399) -> ()  [unwired: 2 in, 2 out]
      }
      event "Calculate Frames": Value Change {
        n176 = event-data() -> ("NewVal"=w409:bool)  [unwired: 1 in, 5 out]
        n177 = case shown="False" w409 {
          tunnel: [0 2] -> w404
          tunnel: w406 -> [w411 w420]
          tunnel: [w411 w418] -> w407
          tunnel: w405 -> [w410 w417]
          tunnel: [w410 w413] -> w403
          frame False {
          }
          frame True {
            w419 = T6 {"QueueAction"=enum."TimeOut", "Numeric 1"=0.0, "Numeric 2"=0.0, "Boolean 1"=FALSE, "Boolean 2"=FALSE, "Spin Program"=[]}  # Device Queue
            n178 = property on="Integration Time" class="DigNum (strict)"() -> ("Value"=w415:dbl[unit])  [unwired: 2 in, 2 out]
            n179 = node(w415) -> (w414:dbl)
            n180 = Bundle By Name(cluster=w419, "QueueAction"=DeviceQueue_Action."Spectrometer_SetIntegrationTime", "Numeric 1"=w414) -> (w421:T6)
            n181 = Enqueue Element(queue=w420, element=w421, error in (no error)=w417) -> (queue out=w418:refnum<queue>, error out=w413:errorcluster)  [unwired: 1 in, 1 out]
          }
        }
        n182 = property on="Frames" class="DigNum (strict)"("DisabledEnum"=w404) -> ()  [unwired: 2 in, 2 out]
      }
      event "Record RefSpec": Value Change {
        w430 = T6 {"QueueAction"=enum."TimeOut", "Numeric 1"=0.0, "Numeric 2"=0.0, "Boolean 1"=FALSE, "Boolean 2"=FALSE, "Spin Program"=[]}  # Device Queue
        n183 = event-data() -> ()  [unwired: 1 in, 6 out]
        n184 = Bundle By Name(cluster=w430, "QueueAction"=DeviceQueue_Action."Spectrometer_SetReference") -> (w429:T6)
        n185 = Enqueue Element(queue=w428, element=w429, error in (no error)=w425) -> (queue out=w426:refnum<queue>, error out=w424:errorcluster)  [unwired: 1 in, 1 out]
      }
      event "Preview": Value Change {
        w438 = T6 {"QueueAction"=enum."TimeOut", "Numeric 1"=0.0, "Numeric 2"=0.0, "Boolean 1"=FALSE, "Boolean 2"=FALSE, "Spin Program"=[]}  # Device Queue
        n186 = event-data() -> ()  [unwired: 1 in, 6 out]
        n187 = Bundle By Name(cluster=w438, "QueueAction"=DeviceQueue_Action."Spectrometer_Preview") -> (w437:T6)
        n188 = Enqueue Element(queue=w435, element=w437, error in (no error)=w433) -> (queue out=w432:refnum<queue>, error out=w431:errorcluster)  [unwired: 1 in, 1 out]
      }
      event "Record_Darkspec": Value Change {
        w446 = T6 {"QueueAction"=enum."TimeOut", "Numeric 1"=0.0, "Numeric 2"=0.0, "Boolean 1"=FALSE, "Boolean 2"=FALSE, "Spin Program"=[]}  # Device Queue
        n189 = event-data() -> ()  [unwired: 1 in, 6 out]
        n190 = Bundle By Name(cluster=w446, "QueueAction"=DeviceQueue_Action."Spectrometer_SetDarkspec") -> (w445:T6)
        n191 = Enqueue Element(queue=w444, element=w445, error in (no error)=w441) -> (queue out=w442:refnum<queue>, error out=w440:errorcluster)  [unwired: 1 in, 1 out]
      }
      event "StartMeasurement_Button": Value Change {
        w453 = T4 {"QueueAction"=enum."TimeOut", "Data"=[], "Data_Raw"=[], "Data_Dark"=[], "Data_Ref"=[], "Device Information"=[], "Numeric Control"=0.0, "Boolean"=FALSE, "Wavelength"=[], "Time"=[], "Time Stamp"=timestamp(0 s since 1904-01-01), "Numeric Control 2"=0.0}  # DataQueue
        w461 = T6 {"QueueAction"=enum."TimeOut", "Numeric 1"=0.0, "Numeric 2"=0.0, "Boolean 1"=FALSE, "Boolean 2"=FALSE, "Spin Program"=[]}  # Device Queue
        n192 = event-data() -> ()  [unwired: 1 in, 6 out]
        n193 = property on="Preview" class="Bool (strict)"("Value"=FALSE ("Preview")) -> ()  [unwired: 2 in, 2 out]
        n194 = Bundle By Name(cluster=w461, "QueueAction"=DeviceQueue_Action."Measure_InSitu") -> (w460:T6)
        n195 = Enqueue Element(queue=w459, element=w460, error in (no error)=w457) -> (queue out=w458:refnum<queue>, error out=w448:errorcluster)  [unwired: 1 in, 1 out]
        n196 = Get Date/Time In Seconds() -> (seconds since 1Jan1904=w447:timestamp)
        n197 = Bundle By Name(cluster=w453, "QueueAction"=DataQueue_Action."Measure_InSituSpinCoating", "Time Stamp"=w447) -> (w454:T4)
        n198 = Enqueue Element(queue=w451, element=w454, error in (no error)=w448) -> (queue out=w450:refnum<queue>, error out=w449:errorcluster)  [unwired: 1 in, 1 out]
      }
      event "StartSpin_Button": Value Change {
        w469 = T6 {"QueueAction"=enum."TimeOut", "Numeric 1"=0.0, "Numeric 2"=0.0, "Boolean 1"=FALSE, "Boolean 2"=FALSE, "Spin Program"=[]}  # Device Queue
        n199 = event-data() -> ()  [unwired: 1 in, 6 out]
        n200 = Bundle By Name(cluster=w469, "QueueAction"=DeviceQueue_Action."Arduino_StartProgram") -> (w468:T6)
        n201 = Enqueue Element(queue=w467, element=w468, error in (no error)=w463) -> (queue out=w465:refnum<queue>, error out=w464:errorcluster)  [unwired: 1 in, 1 out]
      }
      event "Milliseconds": Value Change {
        w478 = T6 {"QueueAction"=enum."TimeOut", "Numeric 1"=0.0, "Numeric 2"=0.0, "Boolean 1"=FALSE, "Boolean 2"=FALSE, "Spin Program"=[]}  # Device Queue
        n202 = event-data() -> ()  [unwired: 1 in, 6 out]
        n203 = Bundle By Name(cluster=w478, "QueueAction"=DeviceQueue_Action."Arduino_SetMillis", "Numeric 1"="Milliseconds") -> (w474:T6)
        n204 = Enqueue Element(queue=w477, element=w474, error in (no error)=w475) -> (queue out=w473:refnum<queue>, error out=w472:errorcluster)  [unwired: 1 in, 1 out]
      }
      event "Speed": Value Change {
        w487 = T6 {"QueueAction"=enum."TimeOut", "Numeric 1"=0.0, "Numeric 2"=0.0, "Boolean 1"=FALSE, "Boolean 2"=FALSE, "Spin Program"=[]}  # Device Queue
        n205 = event-data() -> ()  [unwired: 1 in, 6 out]
        n206 = Bundle By Name(cluster=w487, "QueueAction"=DeviceQueue_Action."Arduino_SetSpeed", "Numeric 1"="Speed") -> (w483:T6)
        n207 = Enqueue Element(queue=w486, element=w483, error in (no error)=w484) -> (queue out=w482:refnum<queue>, error out=w481:errorcluster)  [unwired: 1 in, 1 out]
      }
      event "Debug": Value Change {
        n208 = event-data() -> ()  [unwired: 1 in, 6 out]
        n209 = Select(t=u8 0, s="Debug", f=u8 2) -> (s? t:f=w488:u8)
        n210 = property on="Milliseconds" class="DigNum (strict)"("DisabledEnum"=w488) -> ()  [unwired: 2 in, 2 out]
        n211 = property on="Speed" class="DigNum (strict)"("DisabledEnum"=w488) -> ()  [unwired: 2 in, 2 out]
      }
    }
  }
  n212 = while {
    shift-right: [w499] -> _
    shift-left: w3 -> [w503]
    shift-right: [w500] -> w5
    shift-left: w7 -> [w502]
    shift-right: [w497] -> w4
    shift-left: w2 -> [w498]
    shift-right: [w495] -> _
    shift-left: w6 -> [w496]
    stop <- w501 stop-if-true
    # "Consumer Devices"
    n213 = case shown="No Error" w503 {
      selector: w503 -> [w515 w923]
      tunnel: w502 -> [w516 w924]
      tunnel: [w512 _] -> w501
      tunnel: [w511 w924] -> w500
      tunnel: [w509 w920] -> w499
      tunnel: w498 -> [w507 w918]
      tunnel: [w508 w918] -> w497
      tunnel: w496 -> [w506 w919]
      tunnel: [w505 w919] -> w495
      frame No Error {
        n214 = Dequeue Element(queue=w516, error in (no error)=w515) -> (queue out=w514:refnum<queue>, element=w504:T6, error out=w510:errorcluster)  [unwired: 1 in, 1 out]
        n215 = Unbundle By Name(w504) -> ("QueueAction"=w513:T7)
        n216 = case shown="\"Close_Program\"" w513 {
          tunnel: w514 -> [w520 w540 w546 w555 w604 w618 w625 w655 w662 w681 w687 w717 w740 w761 w771 w783 w795 w806 w822 w824 w831 w847 w860 w871 w907]
          tunnel: [_ w542 _ _ _ _ _ _ _ _ _ _ _ _ _ _ _ _ _ _ _ _ _ _ _] -> w512
          tunnel: [w520 w525 w546 w554 w604 w618 w626 w655 w662 w681 w686 w717 w740 w761 w771 w783 w788 w806 w822 w824 w831 w847 w860 w871 w873] -> w511
          tunnel: w510 -> [w519 w524 w547 w566 w605 w617 w640 w658 w666 w678 w693 w715 w731 w752 w768 w779 w803 w810 w821 w826 w838 w848 w859 w864 w910]
          tunnel: [w519 w523 w545 w553 w599 w616 w627 w656 w663 w668 w685 w714 w730 w751 w766 w773 w787 w809 w817 w825 w832 w846 w855 w863 w874] -> w509
          tunnel: [w517 w522 w550 w551 w601 w613 w634 w654 w661 w672 w695 w718 w723 w744 w762 w775 w801 w808 w819 w830 w842 w844 w861 w866 w872] -> w508
          tunnel: w507 -> [w517 w522 w550 w552 w601 w614 w635 w654 w661 w673 w695 w718 w726 w747 w762 w777 w801 w808 w819 w830 w842 w844 w861 w867 w872]
          tunnel: w506 -> [w518 w521 w549 w563 w603 w615 w624 w653 w665 w674 w684 w711 w722 w743 w765 w772 w800 w807 w818 w829 w841 w843 w858 w865 w912]
          tunnel: [w518 w521 w549 w557 w602 w615 w623 w651 w660 w674 w682 w712 w721 w742 w763 w772 w798 w807 w818 w829 w841 w843 w858 w865 w912] -> w505
          tunnel: w504 -> [_ _ _ _ _ _ _ _ _ w680 w690 w719 _ _ w769 _ _ _ w816 _ w839 w845 _ _ _]
          frame "TimeOut", Default {
          }
          frame "Close_Program" {
            w541 = T6 {"QueueAction"=enum."TimeOut", "Numeric 1"=0.0, "Numeric 2"=0.0, "Boolean 1"=FALSE, "Boolean 2"=FALSE, "Spin Program"=[]}  # Device Queue
            n217 = Bundle By Name(cluster=w541, "QueueAction"=DeviceQueue_Action."Spectrometer_Close") -> (w536:T6)
            n218 = Bundle By Name(cluster=w536, "QueueAction"=DeviceQueue_Action."Laser_Close") -> (w534:T6)
            n219 = Bundle By Name(cluster=w534, "QueueAction"=DeviceQueue_Action."Arduino_Close") -> (w528:T6)
            n220 = Enqueue Element(queue=w540, element=w536, error in (no error)=w524) -> (queue out=w538:refnum<queue>, error out=w533:errorcluster)  [unwired: 1 in, 1 out]
            n221 = Bundle By Name(cluster=w528, "QueueAction"=DeviceQueue_Action."Close_Program") -> (w526:T6)
            n222 = Enqueue Element(queue=w538, element=w534, error in (no error)=w533) -> (queue out=w532:refnum<queue>, error out=w531:errorcluster)  [unwired: 1 in, 1 out]
            n223 = Enqueue Element(queue=w532, element=w528, error in (no error)=w531) -> (queue out=w530:refnum<queue>, error out=w529:errorcluster)  [unwired: 1 in, 1 out]
            n224 = Enqueue Element(queue=w530, element=w526, error in (no error)=w529) -> (queue out=w525:refnum<queue>, error out=w523:errorcluster)  [unwired: 1 in, 1 out]
            n225 = First Call?() -> (First Call?: T/F=w543:bool)
            n226 = Not(x=w543) -> (.not. x?=w542:bool)
          }
          frame "Abort" {
            n227 = Unbundle By Name(w549) -> ("Port Arduino"=w548:refnum<visa-resource-name>)
            n228 = VISA Write(VISA resource name=w548, write buffer="abo", error in (no error)=w547) -> (error out=w545:errorcluster)  [unwired: 2 out]
          }
          frame "Spectrometer_Init" {
            n229 = call-dynamic "Init.vi"("error in (no error)"=w566, "Variant"=0, "Avantes in"=refnum<class "Avantes.lvclass"> refnum ("Avantes.lvclass")) -> ("error out"=w565:errorcluster, "Avantes out"=w564:refnum<class "Avantes.lvclass">)  [unwired: 7 in]
            n230 = call-dynamic "IsInit.vi"("error in (no error)"=w565, "Avantes in"=w564) -> ("error out"=w561:errorcluster, "Is Init?"=w560:bool, "Avantes out"=w562:refnum<class "Avantes.lvclass">)  [unwired: 7 in]
            n231 = property on="Spectromter" class="Bool (strict)"("Value"=w560) -> ()  [unwired: 2 in, 2 out]
            n232 = property on="Init_Spectrometer" class="Bool (strict)"("Value"=w560) -> ()  [unwired: 2 in, 2 out]
            n233 = call-dynamic "Set_ExposurePerFrame.vi"("error in (no error)"=w561, "Exposure per Frame"=1, "Avantes in"=w562) -> ("error out"=w556:errorcluster, "Avantes out"=w559:refnum<class "Avantes.lvclass">)  [unwired: 7 in]
            n234 = case shown="True" w560 {
              tunnel: w559 -> [_ w582]
              tunnel: w556 -> [w571 w580]
              tunnel: [refnum<class "Abstract_CCD.lvclass"> refnum ("Abstract_CCD.lvclass") w581] -> w558
              tunnel: w555 -> [w572 w597]
              tunnel: [w572 w586] -> w554
              tunnel: [w571 w585] -> w553
              tunnel: w552 -> [w570 w577]
              tunnel: [w570 w575] -> w551
              frame False {
              }
              frame True {
                w583 = T4 {"QueueAction"=enum."TimeOut", "Data"=[], "Data_Raw"=[], "Data_Dark"=[], "Data_Ref"=[], "Device Information"=[], "Numeric Control"=0.0, "Boolean"=FALSE, "Wavelength"=[], "Time"=[], "Time Stamp"=timestamp(0 s since 1904-01-01), "Numeric Control 2"=0.0}  # DataQueue
                w598 = T6 {"QueueAction"=enum."TimeOut", "Numeric 1"=0.0, "Numeric 2"=0.0, "Boolean 1"=FALSE, "Boolean 2"=FALSE, "Spin Program"=[]}  # Device Queue
                n235 = call-dynamic "Get_WavelengthAxis.vi"("error in (no error)"=w580, "Avantes in"=w582) -> ("error out"=w579:errorcluster, "lambda"=w574:dbl[unit][], "Avantes out"=w581:refnum<class "Avantes.lvclass">)  [unwired: 7 in]
                n236 = property on="Calculate Frames" class="Bool (strict)"() -> ("Value"=w590:bool)  [unwired: 2 in, 2 out]
                n237 = property on="Integration Time" class="DigNum (strict)"() -> ("Value"=w595:dbl[unit])  [unwired: 2 in, 2 out]
                n238 = Unbundle(w579) -> ("status"=w578:bool)  [unwired: 2 out]
                n239 = node(w595) -> (w594:dbl)
                n240 = Bundle By Name(cluster=w598, "QueueAction"=DeviceQueue_Action."Spectrometer_SetIntegrationTime", "Numeric 1"=w594, "Boolean 1"=w590) -> (w592:T6)
                n241 = property on="Frames" class="DigNum (strict)"() -> ("Value"=w589:i32)  [unwired: 2 in, 2 out]
                n242 = property on="Error_Spectromter" class="Bool (strict)"("Value"=w578) -> ()  [unwired: 2 in, 2 out]
                n243 = Enqueue Element(queue=w597, element=w592, error in (no error)=w580) -> (queue out=w593:refnum<queue>, error out=w587:errorcluster)  [unwired: 1 in, 1 out]
                n244 = Bundle By Name(cluster=w592, "QueueAction"=DeviceQueue_Action."Spectrometer_SetFrames", "Numeric 1"=w589) -> (w588:T6)
                n245 = Bundle By Name(cluster=w583, "QueueAction"=DataQueue_Action."Set_Wavelength", "Wavelength"=w574) -> (w584:T4)
                n246 = Enqueue Element(queue=w577, element=w584) -> (queue out=w575:refnum<queue>)  [unwired: 2 in, 2 out]
                n247 = Enqueue Element(queue=w593, element=w588, error in (no error)=w587) -> (queue out=w586:refnum<queue>, error out=w585:errorcluster)  [unwired: 1 in, 1 out]
              }
            }
            n248 = Bundle By Name(cluster=w563, "Abstract_CCD.lvclass"=w558) -> (w557:T3)
          }
          frame "Spectrometer_Close" {
            n249 = Unbundle By Name(w603) -> ("Abstract_CCD.lvclass"=w606:refnum<class "Abstract_CCD.lvclass">)
            n250 = flat-sequence {
              tunnel: [refnum<class "Abstract_CCD.lvclass"> refnum ("Abstract_CCD.lvclass")] -> w600
              tunnel: w599 -> [_]
              frame #0 {
              }
            }
            n251 = call-dynamic "Close.vi"("error in (no error)"=w605, "Abstract_CCD in"=w606) -> ("error out"=w599:errorcluster)  [unwired: 8 in, 1 out]
            n252 = Bundle By Name(cluster=w603, "Abstract_CCD.lvclass"=w600) -> (w602:T3)
          }
          frame "Spectrometer_Measure" {
            w620 = T4 {"QueueAction"=enum."TimeOut", "Data"=[], "Data_Raw"=[], "Data_Dark"=[], "Data_Ref"=[], "Device Information"=[], "Numeric Control"=0.0, "Boolean"=FALSE, "Wavelength"=[], "Time"=[], "Time Stamp"=timestamp(0 s since 1904-01-01), "Numeric Control 2"=0.0}  # DataQueue
            n253 = Unbundle By Name(w615) -> ("Abstract_CCD.lvclass"=w619:refnum<class "Abstract_CCD.lvclass">)
            n254 = call-dynamic "Measure.vi"("error in (no error)"=w617, "Abstract_CCD in"=w619) -> ("error out"=w616:errorcluster, "Data Raw"=w610:T9, "Data"=w611:T9, "Darkspec"=w609:T9, "Time"=w608:dbl[])  [unwired: 3 in, 2 out]
            n255 = Bundle By Name(cluster=w620, "QueueAction"=DataQueue_Action."TimeOut", "Data"=w611, "Data_Raw"=w610, "Data_Dark"=w609, "Time"=w608) -> (w621:T4)
            n256 = Enqueue Element(queue=w614, element=w621) -> (queue out=w613:refnum<queue>)  [unwired: 2 in, 2 out]
          }
          frame "Spectrometer_Preview" {
            w636 = T4 {"QueueAction"=enum."TimeOut", "Data"=[], "Data_Raw"=[], "Data_Dark"=[], "Data_Ref"=[], "Device Information"=[], "Numeric Control"=0.0, "Boolean"=FALSE, "Wavelength"=[], "Time"=[], "Time Stamp"=timestamp(0 s since 1904-01-01), "Numeric Control 2"=0.0}  # DataQueue
            n257 = Unbundle By Name(w624) -> ("Abstract_CCD.lvclass"=w641:refnum<class "Abstract_CCD.lvclass">)
            n258 = call-dynamic "Get_Frames.vi"("error in (no error)"=w640, "Abstract_CCD in"=w641) -> ("error out"=w642:errorcluster, "Numeric"=w628:i32, "Abstract_CCD out"=w643:refnum<class "Abstract_CCD.lvclass">)  [unwired: 7 in]
            n259 = call-dynamic "Set_Frames.vi"("error in (no error)"=w642, "Frames"=1, "Abstract_CCD in"=w643) -> ("error out"=w639:errorcluster, "Abstract_CCD out"=w644:refnum<class "Abstract_CCD.lvclass">)  [unwired: 7 in]
            n260 = call-dynamic "Measure.vi"("error in (no error)"=w639, "Abstract_CCD in"=w644) -> ("error out"=w630:errorcluster, "Data Raw"=w633:T9, "Abstract_CCD out"=w629:refnum<class "Abstract_CCD.lvclass">)  [unwired: 3 in, 4 out]
            n261 = property on="Preview" class="Bool (strict)"() -> ("Value"=w631:bool)  [unwired: 2 in, 2 out]
            n262 = call-dynamic "Set_Frames.vi"("error in (no error)"=w630, "Frames"=w628, "Abstract_CCD in"=w629) -> ("error out"=w627:errorcluster, "Abstract_CCD out"=w622:refnum<class "Abstract_CCD.lvclass">)  [unwired: 7 in]
            n263 = case shown="True" w631 {
              tunnel: [w645 w647] -> w626
              tunnel: w625 -> [w645 w646]
              frame False {
              }
              frame True {
                w649 = T6 {"QueueAction"=enum."TimeOut", "Numeric 1"=0.0, "Numeric 2"=0.0, "Boolean 1"=FALSE, "Boolean 2"=FALSE, "Spin Program"=[]}  # Device Queue
                n264 = Bundle By Name(cluster=w649, "QueueAction"=DeviceQueue_Action."Spectrometer_Preview") -> (w648:T6)
                n265 = Enqueue Element(queue=w646, element=w648) -> (queue out=w647:refnum<queue>)  [unwired: 2 in, 2 out]
              }
            }
            n266 = Bundle By Name(cluster=w636, "Data_Raw"=w633, "QueueAction"=DataQueue_Action."Spectrometer_Measure") -> (w637:T4)
            n267 = Enqueue Element(queue=w635, element=w637) -> (queue out=w634:refnum<queue>)  [unwired: 2 in, 2 out]
            n268 = Bundle By Name(cluster=w624, "Abstract_CCD.lvclass"=w622) -> (w623:T3)
          }
          frame "Spectrometer_StartMeasurement" {
            n269 = Unbundle By Name(w653) -> ("Abstract_CCD.lvclass"=w657:refnum<class "Abstract_CCD.lvclass">)
            n270 = call-dynamic "StartMeasure.vi"("error in (no error)"=w658, "Frames"=-1, "Abstract_CCD in"=w657) -> ("error out"=w656:errorcluster, "Abstract_CCD out"=w652:refnum<class "Abstract_CCD.lvclass">)  [unwired: 7 in]
            n271 = Bundle By Name(cluster=w653, "Abstract_CCD.lvclass"=w652) -> (w651:T3)
          }
          frame "Spectrometer_StopMeasurement" {
            n272 = Unbundle By Name(w665) -> ("Abstract_CCD.lvclass"=w667:refnum<class "Abstract_CCD.lvclass">)
            n273 = call-dynamic "StopMeasurement.vi"("error in (no error)"=w666, "Abstract_CCD in"=w667) -> ("error out"=w663:errorcluster, "Abstract_CCD out"=w664:refnum<class "Abstract_CCD.lvclass">)  [unwired: 8 in]
            n274 = Bundle By Name(cluster=w665, "Abstract_CCD.lvclass"=w664) -> (w660:T3)
          }
          frame "Spectrometer_GetData" {
            w677 = T4 {"QueueAction"=enum."TimeOut", "Data"=[], "Data_Raw"=[], "Data_Dark"=[], "Data_Ref"=[], "Device Information"=[], "Numeric Control"=0.0, "Boolean"=FALSE, "Wavelength"=[], "Time"=[], "Time Stamp"=timestamp(0 s since 1904-01-01), "Numeric Control 2"=0.0}  # DataQueue
            n275 = Unbundle By Name(w674) -> ("Abstract_CCD.lvclass"=w679:refnum<class "Abstract_CCD.lvclass">)
            n276 = Unbundle By Name(w680) -> ("Numeric 1"=w671:dbl)
            n277 = call-dynamic "Measure_GetData.vi"("error in (no error)"=w678, "SpectraCount"=w671, "Abstract_CCD in"=w679) -> ("error out"=w668:errorcluster, "Data_Raw"=w670:T9, "Time"=w669:dbl[])  [unwired: 5 in, 1 out]
            n278 = Bundle By Name(cluster=w677, "QueueAction"=DataQueue_Action."Spectrometer_Measure", "Data_Raw"=w670, "Time"=w669) -> (w676:T4)
            n279 = Enqueue Element(queue=w673, element=w676) -> (queue out=w672:refnum<queue>)  [unwired: 2 in, 2 out]
          }
          frame "Spectrometer_SetIntegrationTime" {
            n280 = Unbundle By Name(w690) -> ("Numeric 1"=w692:dbl)
            n281 = Unbundle By Name(w684) -> ("Abstract_CCD.lvclass"=w694:refnum<class "Abstract_CCD.lvclass">)
            n282 = Unbundle By Name(w690) -> ("Boolean 1"=w689:bool)
            n283 = node(w692) -> (w691:dbl[unit])
            n284 = call-dynamic "Set_ExposureTime.vi"("error in (no error)"=w693, "Exposure Time"=w691, "Abstract_CCD in"=w694) -> ("error out"=w697:errorcluster, "Abstract_CCD out"=w696:refnum<class "Abstract_CCD.lvclass">)  [unwired: 7 in]
            n285 = call-dynamic "Get_FrameRate.vi"("error in (no error)"=w697, "Abstract_CCD in"=w696) -> ("error out"=w685:errorcluster, "Frame Rate"=w688:dbl[unit], "Abstract_CCD out"=w683:refnum<class "Abstract_CCD.lvclass">)  [unwired: 7 in]
            "Frame Rate" <- w688
            n286 = Bundle By Name(cluster=w684, "Abstract_CCD.lvclass"=w683) -> (w682:T3)
            n287 = case shown="True" w689 {
              tunnel: w688 -> [_ w706]
              tunnel: w687 -> [w698 w700]
              tunnel: [w698 w699] -> w686
              frame False {
              }
              frame True {
                w704 = T6 {"QueueAction"=enum."TimeOut", "Numeric 1"=0.0, "Numeric 2"=0.0, "Boolean 1"=FALSE, "Boolean 2"=FALSE, "Spin Program"=[]}  # Device Queue
                n288 = property on="Program Spin Coater\nSpeed (rpm)          Time (s)" class="Arr (strict)"() -> ("Value"=w709:dbl[][])  [unwired: 2 in, 2 out]
                n289 = property on="Seconds to Spin Start" class="DigNum (strict)"() -> ("Value"=w708:dbl[unit])  [unwired: 2 in, 2 out]
                n290 = property on="Seconds after Spin Stop" class="DigNum (strict)"() -> ("Value"=w707:dbl[unit])  [unwired: 2 in, 2 out]
                n291 = call "CalculateFrames.vi"("Program Spin Coater\nSpeed (rpm)          Time (s)"=w709, "Seconds End"=w707, "Seconds Start"=w708, "Frame Rate"=w706) -> ("Time"=w705:dbl, "Frames"=w701:i32)  [unwired: 6 in]
                n292 = property on="Overall Time" class="DigNum (strict)"("Value"=w705) -> ()  [unwired: 2 in, 2 out]
                n293 = Bundle By Name(cluster=w704, "QueueAction"=DeviceQueue_Action."Spectrometer_SetFrames", "Numeric 1"=w701) -> (w703:T6)
                n294 = Enqueue Element(queue=w700, element=w703) -> (queue out=w699:refnum<queue>)  [unwired: 2 in, 2 out]
              }
            }
          }
          frame "Spectrometer_SetFrames" {
            n295 = Unbundle By Name(w711) -> ("Abstract_CCD.lvclass"=w716:refnum<class "Abstract_CCD.lvclass">)
            n296 = Unbundle By Name(w719) -> ("Numeric 1"=w713:dbl)
            n297 = property on="Frames" class="DigNum (strict)"("Value"=w713) -> ()  [unwired: 2 in, 2 out]
            n298 = call-dynamic "Set_Frames.vi"("error in (no error)"=w715, "Frames"=w713, "Abstract_CCD in"=w716) -> ("error out"=w714:errorcluster, "Abstract_CCD out"=w710:refnum<class "Abstract_CCD.lvclass">)  [unwired: 7 in]
            n299 = Bundle By Name(cluster=w711, "Abstract_CCD.lvclass"=w710) -> (w712:T3)
          }
          frame "Spectrometer_SetDarkspec" {
            w727 = T4 {"QueueAction"=enum."TimeOut", "Data"=[], "Data_Raw"=[], "Data_Dark"=[], "Data_Ref"=[], "Device Information"=[], "Numeric Control"=0.0, "Boolean"=FALSE, "Wavelength"=[], "Time"=[], "Time Stamp"=timestamp(0 s since 1904-01-01), "Numeric Control 2"=0.0}  # DataQueue
            n300 = Unbundle By Name(w722) -> ("Abstract_CCD.lvclass"=w739:refnum<class "Abstract_CCD.lvclass">)
            n301 = property on="Frames for Dark/Ref" class="DigNum (strict)"() -> ("Value"=w729:dbl)  [unwired: 2 in, 2 out]
            n302 = call-dynamic "Get_Frames.vi"("error in (no error)"=w731, "Abstract_CCD in"=w739) -> ("error out"=w736:errorcluster, "Numeric"=w737:i32, "Abstract_CCD out"=w738:refnum<class "Abstract_CCD.lvclass">)  [unwired: 7 in]
            n303 = call-dynamic "Set_Frames.vi"("error in (no error)"=w736, "Frames"=w729, "Abstract_CCD in"=w738) -> ("error out"=w735:errorcluster, "Abstract_CCD out"=w732:refnum<class "Abstract_CCD.lvclass">)  [unwired: 7 in]
            n304 = call-dynamic "Measure.vi"("error in (no error)"=w735, "Abstract_CCD in"=w732) -> ("error out"=w734:errorcluster, "Data Raw"=w724:T9, "Abstract_CCD out"=w733:refnum<class "Abstract_CCD.lvclass">)  [unwired: 3 in, 4 out]
            n305 = call-dynamic "Set_Frames.vi"("error in (no error)"=w734, "Frames"=w737, "Abstract_CCD in"=w733) -> ("error out"=w730:errorcluster, "Abstract_CCD out"=w720:refnum<class "Abstract_CCD.lvclass">)  [unwired: 7 in]
            n306 = Bundle By Name(cluster=w727, "QueueAction"=DataQueue_Action."Set_Dark", "Data_Dark"=w724) -> (w728:T4)
            n307 = Enqueue Element(queue=w726, element=w728) -> (queue out=w723:refnum<queue>)  [unwired: 2 in, 2 out]
            n308 = Bundle By Name(cluster=w722, "Abstract_CCD.lvclass"=w720) -> (w721:T3)
          }
          frame "Spectrometer_SetReference" {
            w748 = T4 {"QueueAction"=enum."TimeOut", "Data"=[], "Data_Raw"=[], "Data_Dark"=[], "Data_Ref"=[], "Device Information"=[], "Numeric Control"=0.0, "Boolean"=FALSE, "Wavelength"=[], "Time"=[], "Time Stamp"=timestamp(0 s since 1904-01-01), "Numeric Control 2"=0.0}  # DataQueue
            n309 = Unbundle By Name(w743) -> ("Abstract_CCD.lvclass"=w760:refnum<class "Abstract_CCD.lvclass">)
            n310 = property on="Frames for Dark/Ref" class="DigNum (strict)"() -> ("Value"=w750:dbl)  [unwired: 2 in, 2 out]
            n311 = call-dynamic "Get_Frames.vi"("error in (no error)"=w752, "Abstract_CCD in"=w760) -> ("error out"=w757:errorcluster, "Numeric"=w758:i32, "Abstract_CCD out"=w759:refnum<class "Abstract_CCD.lvclass">)  [unwired: 7 in]
            n312 = call-dynamic "Set_Frames.vi"("error in (no error)"=w757, "Frames"=w750, "Abstract_CCD in"=w759) -> ("error out"=w756:errorcluster, "Abstract_CCD out"=w753:refnum<class "Abstract_CCD.lvclass">)  [unwired: 7 in]
            n313 = call-dynamic "Measure.vi"("error in (no error)"=w756, "Abstract_CCD in"=w753) -> ("error out"=w755:errorcluster, "Data Raw"=w745:T9, "Abstract_CCD out"=w754:refnum<class "Abstract_CCD.lvclass">)  [unwired: 3 in, 4 out]
            n314 = call-dynamic "Set_Frames.vi"("error in (no error)"=w755, "Frames"=w758, "Abstract_CCD in"=w754) -> ("error out"=w751:errorcluster, "Abstract_CCD out"=w741:refnum<class "Abstract_CCD.lvclass">)  [unwired: 7 in]
            n315 = Bundle By Name(cluster=w748, "QueueAction"=DataQueue_Action."Set_Ref", "Data_Ref"=w745) -> (w749:T4)
            n316 = Enqueue Element(queue=w747, element=w749) -> (queue out=w744:refnum<queue>)  [unwired: 2 in, 2 out]
            n317 = Bundle By Name(cluster=w743, "Abstract_CCD.lvclass"=w741) -> (w742:T3)
          }
          frame "Spectrometer_SetTriggerMode" {
            n318 = Unbundle By Name(w765) -> ("Abstract_CCD.lvclass"=w770:refnum<class "Abstract_CCD.lvclass">)
            n319 = Unbundle By Name(w769) -> ("Numeric 1"=w767:dbl)
            n320 = call-dynamic "Set_TriggerMode.vi"("error in (no error)"=w768, "Trigger Mode"=w767, "Abstract_CCD in"=w770) -> ("error out"=w766:errorcluster, "Abstract_CCD out"=w764:refnum<class "Abstract_CCD.lvclass">)  [unwired: 7 in]
            n321 = Bundle By Name(cluster=w765, "Abstract_CCD.lvclass"=w764) -> (w763:T3)
          }
          frame "Spectrometer_DeviceInformation" {
            w778 = T4 {"QueueAction"=enum."TimeOut", "Data"=[], "Data_Raw"=[], "Data_Dark"=[], "Data_Ref"=[], "Device Information"=[], "Numeric Control"=0.0, "Boolean"=FALSE, "Wavelength"=[], "Time"=[], "Time Stamp"=timestamp(0 s since 1904-01-01), "Numeric Control 2"=0.0}  # DataQueue
            n322 = Unbundle By Name(w772) -> ("Abstract_CCD.lvclass"=w780:refnum<class "Abstract_CCD.lvclass">)
            n323 = call-dynamic "Get_DeviceInformation.vi"("error in (no error)"=w779, "Abstract_CCD in"=w780) -> ("error out"=w774:errorcluster, "Array"=w781:string[])  [unwired: 7 in, 1 out]
            n324 = Bundle By Name(cluster=w778, "QueueAction"=DataQueue_Action."Transfer_Settings", "Device Information"=w781) -> (w776:T4)
            n325 = Enqueue Element(queue=w777, element=w776, error in (no error)=w774) -> (queue out=w775:refnum<queue>, error out=w773:errorcluster)  [unwired: 1 in, 1 out]
          }
          frame "Arduino_Init" {
            w797 = T6 {"QueueAction"=enum."TimeOut", "Numeric 1"=0.0, "Numeric 2"=0.0, "Boolean 1"=FALSE, "Boolean 2"=FALSE, "Spin Program"=[]}  # Device Queue
            n326 = call-poly "VISA Configure Serial Port"("VISA resource name"="Port Arduino", "baud rate (9600)"=u32 115200, "error in (no error)"=w803) -> ("VISA resource name out"=w799:refnum<visa-resource-name>, "error out"=w786:errorcluster)  [unwired: 11 in]
            n327 = Unbundle(w786) -> ("status"=w785:bool)  [unwired: 2 out]
            n328 = Not(x=w785) -> (.not. x?=w784:bool)
            n329 = property on="Arduino" class="Bool (strict)"("Value"=w784) -> ()  [unwired: 2 in, 2 out]
            n330 = property on="Program Spin Coater\nSpeed (rpm)          Time (s)" class="Arr (strict)"() -> ("Value"=w792:dbl[][])  [unwired: 2 in, 2 out]
            n331 = Bundle By Name(cluster=w797, "QueueAction"=DeviceQueue_Action."Arduino_LoadProgram", "Spin Program"=dbl[][] []) -> (w793:T6)
            n332 = Enqueue Element(queue=w795, element=w793, error in (no error)=w786) -> (queue out=w791:refnum<queue>, error out=w790:errorcluster)  [unwired: 1 in, 1 out]
            n333 = Bundle By Name(cluster=w793, "Spin Program"=w792) -> (w789:T6)
            n334 = Bundle By Name(cluster=w800, "Port Arduino"=w799) -> (w798:T3)
            n335 = Enqueue Element(queue=w791, element=w789, error in (no error)=w790) -> (queue out=w788:refnum<queue>, error out=w787:errorcluster)  [unwired: 1 in, 1 out]
          }
          frame "Arduino_Close" {
            n336 = Unbundle By Name(w807) -> ("Port Arduino"=w811:refnum<visa-resource-name>)
            n337 = property on="Arduino" class="Bool (strict)"("Value"=FALSE ("Arduino")) -> ()  [unwired: 2 in, 2 out]
            n338 = VISA Close(VISA resource name=w811, error in (no error)=w810) -> (error out=w809:errorcluster)
          }
          frame "Arduino_LoadProgram" {
            n339 = Unbundle By Name(w816) -> ("Spin Program"=w815:dbl[][], "Numeric 1"=w813:dbl)
            n340 = Unbundle By Name(w818) -> ("Port Arduino"=w820:refnum<visa-resource-name>)
            n341 = node(w813) -> (w812:dbl[unit])
            n342 = call "SpinCoaterArray2String_v02.vi"("Time Start"=w812, "Program Spin Coater\nSpeed (rpm)          Time (s)"=w815) -> ("remote control String"=w814:string)  [unwired: 3 in]
            n343 = VISA Write(VISA resource name=w820, write buffer=w814, error in (no error)=w821) -> (error out=w817:errorcluster)  [unwired: 2 out]
          }
          frame "Arduino_StartProgram" {
            n344 = Unbundle By Name(w829) -> ("Port Arduino"=w828:refnum<visa-resource-name>)
            n345 = VISA Write(VISA resource name=w828, write buffer="run", error in (no error)=w826) -> (error out=w825:errorcluster)  [unwired: 2 out]
            n346 = property on="Action" class="Str"("Value"="Measuring" ("Action")) -> ()  [unwired: 2 in, 2 out]
          }
          frame "Arduino_SetSpeed" {
            n347 = Unbundle By Name(w839) -> ("Numeric 1"=w837:dbl)
            n348 = Unbundle By Name(w841) -> ("Port Arduino"=w840:refnum<visa-resource-name>)
            n349 = To Unsigned Long Integer(number=w837) -> (unsigned 32bit integer=w836:u32)
            n350 = Number To Decimal String(number=w836) -> (decimal integer string=w835:string)  [unwired: 1 in]
            n351 = Concatenate Strings("!spe" ("string"), w835) -> (w833:string)
            n352 = VISA Write(VISA resource name=w840, write buffer=w833, error in (no error)=w838) -> (error out=w832:errorcluster)  [unwired: 2 out]
          }
          frame "Arduino_SetMillis" {
            n353 = Unbundle By Name(w845) -> ("Numeric 1"=w853:dbl)
            n354 = Unbundle By Name(w843) -> ("Port Arduino"=w854:refnum<visa-resource-name>)
            n355 = To Unsigned Long Integer(number=w853) -> (unsigned 32bit integer=w852:u32)
            n356 = Number To Decimal String(number=w852) -> (decimal integer string=w851:string)  [unwired: 1 in]
            n357 = Concatenate Strings("!mil" ("string"), w851) -> (w849:string)
            n358 = VISA Write(VISA resource name=w854, write buffer=w849, error in (no error)=w848) -> (error out=w846:errorcluster)  [unwired: 2 out]
          }
          frame "Arduino_StopSpin" {
            n359 = Unbundle By Name(w858) -> ("Port Arduino"=w857:refnum<visa-resource-name>)
            n360 = VISA Write(VISA resource name=w857, write buffer="abo", error in (no error)=w859) -> (error out=w855:errorcluster)  [unwired: 2 out]
          }
          frame "Measure_Stop" {
            w869 = T4 {"QueueAction"=enum."TimeOut", "Data"=[], "Data_Raw"=[], "Data_Dark"=[], "Data_Ref"=[], "Device Information"=[], "Numeric Control"=0.0, "Boolean"=FALSE, "Wavelength"=[], "Time"=[], "Time Stamp"=timestamp(0 s since 1904-01-01), "Numeric Control 2"=0.0}  # DataQueue
            n361 = Bundle By Name(cluster=w869, "QueueAction"=DataQueue_Action."Stop_Measurement") -> (w870:T4)
            n362 = Enqueue Element(queue=w867, element=w870, error in (no error)=w864) -> (queue out=w866:refnum<queue>, error out=w863:errorcluster)  [unwired: 1 in, 1 out]
            n363 = property on="StartMeasurement_Button" class="Bool (strict)"("Value"=FALSE ("StartMeasurement_Button")) -> ()  [unwired: 2 in, 2 out]
          }
          frame "Measure_InSitu" {
            w884 = 1000 ("y")
            w900 = T6 {"QueueAction"=enum."TimeOut", "Numeric 1"=0.0, "Numeric 2"=0.0, "Boolean 1"=FALSE, "Boolean 2"=FALSE, "Spin Program"=[]}  # Device Queue
            w908 = T6 {"QueueAction"=enum."TimeOut", "Numeric 1"=0.0, "Numeric 2"=0.0, "Boolean 1"=FALSE, "Boolean 2"=FALSE, "Spin Program"=[]}  # Device Queue
            n364 = Unbundle By Name(w912) -> ("Abstract_CCD.lvclass"=w911:refnum<class "Abstract_CCD.lvclass">)
            n365 = call-dynamic "Get_Frames.vi"("error in (no error)"=w910, "Abstract_CCD in"=w911) -> ("error out"=w905:errorcluster, "Numeric"=w895:i32)  [unwired: 7 in, 1 out]
            n366 = Bundle By Name(cluster=w908, "QueueAction"=DeviceQueue_Action."Spectrometer_SetTriggerMode", "Numeric 1"=1.0) -> (w906:T6)
            n367 = Bundle By Name(cluster=w900, "QueueAction"=DeviceQueue_Action."Spectrometer_DeviceInformation") -> (w897:T6)
            n368 = Bundle By Name(cluster=w897, "QueueAction"=DeviceQueue_Action."Spectrometer_StartMeasurement") -> (w892:T6)
            n369 = Enqueue Element(queue=w907, element=w906, error in (no error)=w905) -> (queue out=w902:refnum<queue>, error out=w903:errorcluster)  [unwired: 1 in, 1 out]
            n370 = Bundle By Name(cluster=w892, "QueueAction"=DeviceQueue_Action."Arduino_StartProgram") -> (w887:T6)
            n371 = Enqueue Element(queue=w902, element=w897, error in (no error)=w903) -> (queue out=w899:refnum<queue>, error out=w898:errorcluster)  [unwired: 1 in, 1 out]
            n372 = Bundle By Name(cluster=w887, "QueueAction"=DeviceQueue_Action."Spectrometer_GetData", "Numeric 1"=w884) -> (w881:T6)
            n373 = Divide(x=w895, y=w884) -> (x/y=w894:dbl)
            n374 = Round Toward +Infinity(x=w894) -> (ceil(x): smallest int >= x=w893:dbl)
            n375 = Enqueue Element(queue=w899, element=w892, error in (no error)=w898) -> (queue out=w891:refnum<queue>, error out=w890:errorcluster)  [unwired: 1 in, 1 out]
            n376 = Enqueue Element(queue=w891, element=w887, error in (no error)=w890) -> (queue out=w888:refnum<queue>, error out=w885:errorcluster)  [unwired: 1 in, 1 out]
            n377 = for {
              N: w893 -> [_]
              shift-right: [w913] -> w883
              shift-left: w888 -> [w917]
              tunnel: w881 -> [w914]
              shift-right: [w915] -> w882
              shift-left: w885 -> [w916]
              n378 = Enqueue Element(queue=w917, element=w914, error in (no error)=w916) -> (queue out=w913:refnum<queue>, error out=w915:errorcluster)  [unwired: 1 in, 1 out]
            }
            n379 = Bundle By Name(cluster=w881, "QueueAction"=DeviceQueue_Action."Spectrometer_StopMeasurement") -> (w877:T6)
            n380 = Bundle By Name(cluster=w877, "QueueAction"=DeviceQueue_Action."Measure_Stop") -> (w875:T6)
            n381 = Enqueue Element(queue=w883, element=w877, error in (no error)=w882) -> (queue out=w878:refnum<queue>, error out=w879:errorcluster)  [unwired: 1 in, 1 out]
            n382 = Enqueue Element(queue=w878, element=w875, error in (no error)=w879) -> (queue out=w873:refnum<queue>, error out=w874:errorcluster)  [unwired: 1 in, 1 out]
          }
        }
      }
      frame Error {
        w922 = T12 4 items=["no dialog", "OK message", "continue or stop message", "OK message + warnings", "continue/stop + warnings"] ("type of dialog (OK msg:1)")
        n383 = call <vilib>:"General Error Handler.vi"("type of dialog (OK msg:1)"=w922, "error in (no error)"=w923) -> ("error out"=w921:errorcluster)  [unwired: 9 in, 4 out]
        n384 = call <vilib>:"Clear Errors.vi"("error in (no error)"=w921) -> ("error out"=w920:errorcluster)  [unwired: 5 in, 1 out]
      }
    }
  }
  n385 = Release Queue(queue=w4) -> ()  [unwired: 2 in, 3 out]
  n386 = Release Queue(queue=w5) -> ()  [unwired: 2 in, 3 out]
